vi "ProfilerTest.vi"() -> ()   [LabVIEW 2014]
uses:
  <vilib>/gmath/NI_Gmath.lvlib
panel:
  out "PositionProfile":cluster{cluster{dbl, dbl}[]}[](graph)=[{[{0.3585789582402244, 0.0}, {0.36140732971089534, -5.036567638092828e-07}, {0.36423581606672245, -9.61293257835823e-07}, {0.3670642302197405, -1.2546678051931824e-06}, {0.369892391773747, -1.1873323667103292e-06}, {0.3727209906863886, -4.852288259001522e-07}, {0.3755493268961446, 1.2019361819159102e-06}, {0.37837772838603073, 4.299709065192369e-06}, {0.38120612229890677, 9.306861087923713e-06}, {0.3840346937672675, 1.6794161055370797e-05}, {0.38686309715876277, 2.7400089421020022e-05}, {0.38969142959159164, 4.1830568179446516e-05}, {0.3925198402830219, 6.085616643129184e-05}, {0.39534837283852375, 8.530833036253735e-05}, {0.3981769428965464, 0.00011607503881997503}, {0.40100531487252966, 0.00015409536549003676}, {0.4038337851980858, 0.0002003653925144592}, {0.4066620491729108, 0.0002559183910066756}, {0.40949064017475745, 0.00032184661067566995}, {0.41231898267404327, 0.0003992561626145476}, {0.4151472322459584, 0.0004893018031565737}, {0.4179757913643334, 0.0005931795898988288}, {0.42080424013440515, 0.0007120817475880187}, {0.42363261299972726, 0.0008472339924668812}, {0.4264611387688061, 0.0009998885386174}, {0.42928945496510473, 0.0011712756792556854}, {0.4321180300590645, 0.0013626797839679785}, {0.4349463962629788, 0.0015753251147018839}, {0.43777465022828593, 0.0018104656195099959}, {0.4406032226432617, 0.0020693801641639095}, {0.4434315120502036, 0.0023532398256405924}, {0.44626009279999124, 0.0026633085947595217}, {0.4490885496571133, 0.0030007250958818303}, {0.4519170062439872, 0.0033666550409679917}, {0.45474539180496276, 0.0037622072978145747}, {0.4575737400814671, 0.004188465921919652}, {0.4604023558724684, 0.00464651952063507}, {0.4632306508066975, 0.005137264322612427}, {0.4660590176954227, 0.0056617062591942675}, {0.46888754518422093, 0.006220754083531697}, {0.47171598682256316, 0.006815191097196341}, {0.47454419326877034, 0.007445749606160159}, {0.47737285109456384, 0.008113292873994857}, {0.4802013404974829, 0.008818319578063984}, {0.4830295733801785, 0.0095613694727503}, {0.48585812789442756, 0.010343094603175375}, {0.48868640379899964, 0.011163755381214013}, {0.4915149544924278, 0.012023862733814084}, {0.49434329506372604, 0.012923544535122886}, {0.497171737305647, 0.013863094164634368}, {0.5000002749584594, 0.014842631910283946}, {0.5028286305191115, 0.015862099281043703}, {0.5056569781980829, 0.016921515585541176}, {0.5084855530715745, 0.018020855308149553}, {0.5113138558379144, 0.019159726963599216}, {0.5141422566436455, 0.020338001953235096}, {0.5169706346971762, 0.021555281125875562}, {0.5197992068851479, 0.022811235874616413}, {0.5226275593510029, 0.02410518309111191}, {0.5254560377756676, 0.025436708787521183}, {0.528284286027275, 0.026805003940692}, {0.5311127926252351, 0.02820959945311543}, {0.5339412791135189, 0.029649591762413142}, {0.5367697939830852, 0.031124175019706785}, {0.5395980099037839, 0.032632285569350675}, {0.5424265819503729, 0.03417333154853474}, {0.545255072269434, 0.03574608666415281}, {0.5480834517870963, 0.03734949267315463}, {0.5509118902564176, 0.03898256385355613}, {0.553740368824329, 0.04064417171967369}, {0.556568652677063, 0.04233302336120809}, {0.5593971125961626, 0.044048158165816725}, {0.5622256826953395, 0.04578833390525411}, {0.5650541408427635, 0.047552188047106835}, {0.5678823695638735, 0.04933840260698288}, {0.5707107335249578, 0.051145956448161785}, {0.5735393080219774, 0.05297364612388425}, {0.5763678204221673, 0.054820041534700194}, {0.5791962794223798, 0.05668389668842144}, {0.5820244134875872, 0.05856378880205473}, {0.5848531114955801, 0.06045908490205213}, {0.5876815198777922, 0.06236800907963759}, {0.590509811808415, 0.0642894935472419}, {0.5933381994308217, 0.06622252965639741}, {0.5961666861819129, 0.06816600181322202}, {0.5989949592951849, 0.07011861347290503}, {0.6018236974459827, 0.07207979542981183}, {0.6046518706223064, 0.07404784077762908}, {0.6074804451692932, 0.07602247913536116}, {0.6103087856472974, 0.07800237936364145}, {0.6131370939005591, 0.0799868514455843}, {0.6159655299441653, 0.08197523809866301}, {0.6187940939091453, 0.08396683389452729}, {0.6216224220212786, 0.08596074317195565}, {0.6244511272184643, 0.08795682791272567}, {0.6272792419089648, 0.08995390636154527}, {0.6301078589095738, 0.09195232466329135}, {0.6329362560771964, 0.09395122235875845}, {0.6357645981270923, 0.09595044178684581}, {0.6385932589450429, 0.0979500507769548}, {0.6414214187260036, 0.09994935160113598}, {1.6313712381539545, 0.7999493516011359}, {1.6370281665398847, 0.803951419959496}, {1.642684574332719, 0.8079529359236688}, {1.6483415120027398, 0.8119541698494368}, {1.6539983690163287, 0.8159539039077326}, {1.6596556635054802, 0.819951408197701}, {1.6653125310660257, 0.8239446701543608}, {1.6709694703145168, 0.8279323401920422}, {1.6766263531941783, 0.8319123326675287}, {1.682282985074101, 0.8358822305251936}, {1.6879394068533564, 0.8398395066604479}, {1.6935964190626638, 0.8437818960051781}, {1.6992532184268627, 0.8477057580086892}, {1.70491063008667, 0.8516083400146843}, {1.7105670391496792, 0.8554849779734043}, {1.7162237784800585, 0.859332821530174}, {1.7218811935075897, 0.8631481275702646}, {1.7275374178826466, 0.8669254871798622}, {1.7331945304300687, 0.870661967100665}, {1.7388514364958167, 0.8743523602708978}, {1.744508275250376, 0.8779921498769128}, {1.7501653995857358, 0.8815768325883049}, {1.7558217882719545, 0.8851009438527649}, {1.7614788664277674, 0.8885604691316429}, {1.767135829491985, 0.8919499440861656}, {1.772792234930327, 0.8952641148568315}, {1.7784493026829933, 0.8984986725061798}, {1.7841064026905955, 0.9016482200345362}, {1.7897632647477684, 0.9047076096157937}, {1.795420199823116, 0.9076720509463055}, {1.80107684483402, 0.9105364564236967}, {1.806733525727416, 0.9132961736478062}, {1.812390409338302, 0.9159465504697608}, {1.8180473081359514, 0.918482881798126}, {1.82370424507416, 0.920900699672133}, {1.8293609976576792, 0.9231955892377075}, {1.8350178638388264, 0.9253635183875473}, {1.8406748547831566, 0.9274005134168232}, {1.8463319774832216, 0.929302798916601}, {1.851988344019988, 0.9310665464586092}, {1.8576452637076741, 0.932688849389749}, {1.8633020150717972, 0.9341664072216153}, {1.8689588347334438, 0.9354964617036569}, {1.874615856039072, 0.9366764760483167}, {1.8802726191382602, 0.9377040757084186}, {1.885929833727203, 0.9385773862648643}, {1.8915861462936545, 0.9392945155796241}, {1.8972436746684436, 0.939854317274878}, {1.9028999138372154, 0.9402554507202174}, {1.9085569721805382, 0.9404972992417304}, {1.9142139634722453, 0.9405793203438549}, {1.9198707247573814, 0.9405013664325429}, {1.9255274979690329, 0.9402636012217233}, {1.9311844809276448, 0.9398664798144253}, {1.9368416418874643, 0.9393107740797157}, {1.9424982407207014, 0.9385976688034054}, {1.948154770427408, 0.9377285296837929}, {1.9538118311419879, 0.9367049472413911}, {1.959468704245492, 0.935529032771663}, {1.9651257500661143, 0.9342029930217137}, {1.9707824942395522, 0.9327295017555716}, {1.9764394982683444, 0.9311112384142088}, {1.9820960133629753, 0.9293515049839838}, {1.987753292494381, 0.9274532241336241}, {1.9934099090348023, 0.9254204232738688}, {1.99906686783999, 0.9232565214374397}, {2.0047237967048193, 0.9209656200506127}, {2.010380279393679, 0.9185520585915949}, {2.0160374263955583, 0.9160196807400908}, {2.0216939973209773, 0.9133735151338472}, {2.027350721004126, 0.910617844173485}, {2.0330078033969303, 0.9077572799132123}, {2.038664652777534, 0.904796942768744}, {2.0443217038394996, 0.9017415095326125}, {2.049978713640327, 0.8985960699865745}, {2.0556351461826123, 0.8953659381838422}, {2.0612919670827305, 0.892055588232734}, {2.066949166324256, 0.8886700317323528}, {2.072606042851228, 0.8852146891765559}, {2.0782628300431796, 0.8816943878809597}, {2.083919355872701, 0.8781141434552929}, {2.089576718776267, 0.8744780766014809}, {2.095233186517815, 0.8707920282241328}, {2.1008897971805096, 0.86705994231616}, {2.1065466194975815, 0.8632862453826441}, {2.1122035140675552, 0.8594753517073581}, {2.117860350300693, 0.8556315044422685}, {2.1235176422115813, 0.8517583212002827}, {2.129174356576727, 0.8478602789857945}, {2.1348312426096725, 0.8439404168465451}, {2.1404879039373634, 0.8400023320094359}, {2.146144651193938, 0.8360488879988732}, {2.151801616247107, 0.8320828154025052}, {2.157458635116028, 0.8281067859203439}, {2.1631152363361923, 0.8241234126529265}, {2.1687724668390422, 0.8201339534180261}, {2.174428903431, 0.8161411137841654}, {2.1800862117160427, 0.8121451197611759}, {2.185743088670165, 0.8081479874562176}, {2.1913996477159907, 0.8041504229032101}, {2.1970564563934145, 0.8001524978094131}, {3.1870059092933873, 0.10015249780941327}, {3.189834376952661, 0.09815196485448308}, {3.1926628208961687, 0.09615149471398858}, {3.195491154710077, 0.09415126670604042}, {3.198319814247035, 0.09215116912790172}, {3.2011480562768933, 0.09015200147095218}, {3.203976421854729, 0.08815373158884615}, {3.2068048663805646, 0.08615681655403101}, {3.2096333044469065, 0.08416181555271954}, {3.2124617645743654, 0.08216927872519217}, {3.215290160671209, 0.08017990602938493}, {3.2181187577501067, 0.07819421736052339}, {3.220946939449224, 0.07621341471380688}, {3.2237754858940275, 0.07423778222708795}, {3.22660380801813, 0.07226861983350559}, {3.2294323811680914, 0.07030653890209591}, {3.2322606991785543, 0.06835288293881592}, {3.2350893436336823, 0.0664082894900329}, {3.237917517860741, 0.06447438652101888}, {3.240745929431053, 0.06255180797125205}, {3.243574513512423, 0.06064175320269017}, {3.2464029865024893, 0.058745595987286174}, {3.249231234621287, 0.05686461618439337}, {3.2520597500573265, 0.05499971257506911}, {3.2548881873074937, 0.053152355156413957}, {3.25771668038416, 0.051323706706228676}, {3.260545012761648, 0.04951516151427515}, {3.2633734499117364, 0.04772780461430523}, {3.266201939035123, 0.04596292162031383}, {3.269030408345825, 0.04422179831825756}, {3.2718586604861892, 0.0425057788627582}, {3.2746872201396093, 0.040815752293008385}, {3.2775155378570093, 0.03915322950542233}, {3.280344045893975, 0.037519108419200184}, {3.28317252049387, 0.03591463984025024}, {3.2860008019498648, 0.03434099182862359}, {3.2888292025282784, 0.03279902820106029}, {3.291657898402663, 0.0312896524823099}, {3.2944861081495787, 0.029814220407712727}, {3.297314487927476, 0.02837327209971384}, {3.3001430356348505, 0.026967645470529503}, {3.302971545797128, 0.025598214957484447}, {3.305800015690742, 0.024265686411860637}, {3.308628313751244, 0.02297075698372346}, {3.311456837717748, 0.021713815872416345}, {3.3142851063333936, 0.02049557511542688}, {3.317113510341176, 0.01931628938178402}, {3.319942140639503, 0.018176278701657805}, {3.322770475473191, 0.017076025894279714}, {3.325598951730509, 0.0160155542477583}, {3.3284271585701153, 0.014995133269844946}, {3.331255650673881, 0.014014602610481333}, {3.3340842016902306, 0.013074008573941046}, {3.3369126832522826, 0.012173275404529102}, {3.3397410238060945, 0.011312224954167158}, {3.342569505843347, 0.010490497226123927}, {3.3453979692051306, 0.00970779087551378}, {3.348226168550258, 0.008963742531939212}, {3.3510547303200977, 0.00825769055905251}, {3.3538831373264912, 0.007589198022618135}, {3.356711646823256, 0.006957563668547689}, {3.359539843986255, 0.0063621701239242046}, {3.362368579114789, 0.005802072774378289}, {3.365196907570558, 0.005276630500459872}, {3.3680251947372883, 0.004784879138177739}, {3.3708538439069944, 0.00432581205227503}, {3.37368212832295, 0.00389855473132987}, {3.3765105999367697, 0.00350198195863069}, {3.3793390609903295, 0.0031350432068672773}, {3.382167341786597, 0.002796638458215678}, {3.384995900625516, 0.0024855615832211353}, {3.387824100002938, 0.0022006998955641788}, {3.3906525370972926, 0.001940785463632702}, {3.3934812447082754, 0.0017045960409560468}, {3.396309623342623, 0.0014909403278989125}, {3.399138009814577, 0.0012985386143856414}, {3.401966239444692, 0.0011261452085499501}, {3.404794884911576, 0.0009724724544487723}, {3.4076233428838814, 0.0008363048810501872}, {3.4104517350040227, 0.0007163937146592025}, {3.413279971886032, 0.0006115152322606204}, {3.416108674337413, 0.0005204426005797208}, {3.418937066744051, 0.00044202012932857693}, {3.4217652592109435, 0.00037508878451707195}, {3.424593666374727, 0.0003185198239412934}, {3.427422277158417, 0.00027123457375897997}, {3.4302507673102225, 0.0002321999436666472}, {3.4330789383343356, 0.0002004244303096675}, {3.4359075310972456, 0.00017495792053558168}, {3.4387360868980017, 0.00015491760982501435}, {3.441564460491389, 0.00013947326521591974}, {3.4443927904586418, 0.00012785381448950084}, {3.4472212072183313, 0.00011935286022231317}, {3.4500497082942103, 0.00011333131431554011}, {3.45287823807302, 0.00010921918252003449}, {3.4557064000578945, 0.00010651794748479937}, {3.458534865041683, 0.00010480148475842943}, {3.461363484864872, 0.00010371967740131771}, {3.464191891692424, 0.000102998649759517}, {3.4670201802152696, 0.00010244185295481267}, {3.469848696679472, 0.00010193103453323693}]}, {[{-0.19999989876479196, 0.0}, {-0.19599968101011692, -1.0073890062435072e-06}, {-0.19199994667744594, -1.9225945871386622e-06}, {-0.18799999265754622, -2.5093928300131422e-06}, {-0.1839997845362129, -2.374731211715307e-06}, {-0.17999974440499977, -9.705808353379095e-07}, {-0.17599979749828915, 2.403802486573782e-06}, {-0.17199988165080565, 8.599268291656234e-06}, {-0.16799989365427387, 1.8613647522725885e-05}, {-0.16399974641027576, 3.3588001121278266e-05}, {-0.1599997925054006, 5.4799691746145115e-05}, {-0.15599971752805983, 8.366224932173939e-05}, {-0.1519999497491696, 0.00012171155347277046}, {-0.14799969116464354, 0.00017061719927788325}, {-0.14399969044576694, 0.00023214732640653593}, {-0.13999981710696696, 0.00030818635937504747}, {-0.13599971002251018, 0.00040072669020160844}, {-0.13199972051983241, 0.0005118385846248636}, {-0.12799954398961128, 0.0006436933966885023}, {-0.12399969135950169, 0.0007985113946655726}, {-0.11999953380714436, 0.0009786223206733522}, {-0.11599977635493537, 0.0011863568434762873}, {-0.11199968221715566, 0.0014241648800392122}, {-0.1079995336266278, 0.0016944857648968758}, {-0.1039995400032736, 0.001999785318751084}, {-0.0999995485779444, 0.0023425740446704636}, {-0.09599988630439422, 0.002725329666204823}, {-0.09199964994606155, 0.003150653182229347}, {-0.0879995735663378, 0.003620974170090313}, {-0.08399980405477737, 0.004138748410156852}, {-0.07999999916436557, 0.004706466584627505}, {-0.0759998629865118, 0.005326589855729003}, {-0.07199961765286897, 0.006001456251807512}, {-0.06799979603645853, 0.006733274802642866}, {-0.06399986297303943, 0.007524374874632924}, {-0.05999988752456636, 0.008376908350246326}, {-0.05599990000907039, 0.009292947639581864}, {-0.05199983599363788, 0.01027449455001387}, {-0.0479997168866717, 0.011323431486463826}, {-0.043999880594600596, 0.012441440279665605}, {-0.03999975405466372, 0.013630342589506319}, {-0.0359996009332965, 0.014891608226232011}, {-0.0319998496375525, 0.016226503794618343}, {-0.027999840689221626, 0.017636524080817256}, {-0.023999769484300045, 0.01912274965632081}, {-0.019999859236598534, 0.02068609238390031}, {-0.015999581163923807, 0.022327615932514405}, {-0.011999560949191997, 0.024047767634961383}, {-0.007999627735662542, 0.0258471587522783}, {-0.003999840056932571, 0.027726148951964028}, {4.1224803332798345e-08, 0.029685085391621735}, {0.004000050239789517, 0.031724070314499614}, {0.008000456453749596, 0.03384317789924717}, {0.012000279308808297, 0.036041646730799924}, {0.01600045667166006, 0.03831959245048956}, {0.020000319536075086, 0.0406760872990872}, {0.024000111618094132, 0.043110562715697}, {0.028000225990225294, 0.04562241437367817}, {0.032000049999004576, 0.048210260902798945}, {0.03600008512101396, 0.0508732840581242}, {0.04000039271398916, 0.05361025939014283}, {0.044000091642358304, 0.05641916285666922}, {0.048000181014672, 0.059299150534354306}, {0.05200011351256987, 0.062248173384726865}, {0.056000112327799806, 0.06526461734444017}, {0.06000022144401757, 0.06834663565227124}, {0.064000383055079, 0.07149220267414197}, {0.06800031247824058, 0.07469901258558052}, {0.07200034033342433, 0.07796516512426935}, {0.07600027932901354, 0.08128826939114384}, {0.08000026425003828, 0.08466613105003873}, {0.0840001923497527, 0.08809629967990842}, {0.0880003922731866, 0.09157664885847029}, {0.0920002782494199, 0.0951042166523484}, {0.09600047961452424, 0.09867707678906977}, {0.10000000532914792, 0.10229183759674812}, {0.10400001306758956, 0.10594703169374545}, {0.10800036848861945, 0.1096400376566363}, {0.11200032981283371, 0.11336766901734488}, {0.11600008949348195, 0.11712761642391986}, {0.12000007493219605, 0.12091783055886571}, {0.12400034372560143, 0.1247359592065738}, {0.12800032101307562, 0.1285790899697627}, {0.13200010382857721, 0.1324450062315782}, {0.136000282340795, 0.136332041830554}, {0.140000107015834, 0.1402373066816576}, {0.14400010015815898, 0.14415923185061982}, {0.14800022290551634, 0.14809579610572363}, {0.15200043336748306, 0.15204507487706104}, {0.15600046519792107, 0.15600502838951402}, {0.16000030990992947, 0.15997398560380838}, {0.16400028639019507, 0.16395072318406365}, {0.16800034270890934, 0.16793377813693242}, {0.17200018742098142, 0.1719215813066752}, {0.17600029908556936, 0.1759134694582433}, {0.18000030977545484, 0.17990807800480932}, {0.18400043689948456, 0.18390477310907577}, {0.18800042429414585, 0.18790259797400644}, {0.19200038479082773, 0.1919011173282485}, {0.19600040771091862, 0.1959000275178594}, {0.20000004677832364, 0.19989864599950807}, {0.4414214002333889, 0.44132000223681755}, {0.4425930563548353, 0.44249174477995745}, {0.44376451083174406, 0.44366327776622694}, {0.4449361528206526, 0.44483497009649164}, {0.44610773574002566, 0.4460065414606963}, {0.4472792694650633, 0.44717795473398797}, {0.4484508146081704, 0.4483492104091164}, {0.4496225058954555, 0.44952037013522933}, {0.4507940466763791, 0.450691051809895}, {0.45196552872069967, 0.4518612494012046}, {0.45313714814505635, 0.45303104906957864}, {0.45430870800618584, 0.4542001329972505}, {0.455480368486206, 0.4553685288935537}, {0.4566518320526547, 0.45653579765596497}, {0.4578234266226369, 0.45770211372784}, {0.45899499073062155, 0.45886715458815225}, {0.4601665696585886, 0.46003079501259997}, {0.4613382066626694, 0.4611928995789317}, {0.46250980465709973, 0.4623531864472321}, {0.4636813333148966, 0.46351143382539056}, {0.46485294696082025, 0.4646675964660735}, {0.46602440998324857, 0.46582123931988156}, {0.4671960103661306, 0.46697243909305663}, {0.4683675673018719, 0.4681208075153042}, {0.4695392113563284, 0.4692662595439}, {0.4707106821148058, 0.47040832639914043}, {0.4718822981449211, 0.4715471033725848}, {0.47305394571359355, 0.4726822637245265}, {0.4742254015820826, 0.47381337739933127}, {0.475397014001019, 0.4749405679832672}, {0.4765685434857642, 0.4760633943946943}, {0.47774024306100515, 0.4771818916827408}, {0.47891171261257387, 0.47829547550435225}, {0.480083269082721, 0.4794042502387827}, {0.4812549326403847, 0.480508041729458}, {0.4824264162590043, 0.48160639457731486}, {0.4835980290984438, 0.4826994207461059}, {0.48476959934296643, 0.4837867890638945}, {0.48594119639124184, 0.48486840240009016}, {0.4871127014588357, 0.48594399920929526}, {0.4882843839237273, 0.48701368363768904}, {0.48945586984689426, 0.4880769823776956}, {0.4906274495843984, 0.4891340386619428}, {0.49179905695308623, 0.49018468209207416}, {0.4929705646527205, 0.4912287012783078}, {0.49414213910265375, 0.4922661592233995}, {0.4953137471707906, 0.493296952737306}, {0.4964853379325727, 0.4943209767511561}, {0.4976569412605734, 0.49533821040362036}, {0.49882846385056656, 0.4963485395687738}, {0.5000001007577792, 0.49735211188887296}, {0.5011717107493813, 0.49834879885449046}, {0.5023431819019044, 0.4993385134777973}, {0.503514804291589, 0.5003215210017554}, {0.5046863878897527, 0.5012976947188631}, {0.5058578771874219, 0.5022670365425134}, {0.507029449302316, 0.5032297532462725}, {0.5082010843849928, 0.5041859002731838}, {0.5093726385054977, 0.5051354459039696}, {0.5105441823005161, 0.5060785459842273}, {0.5117158470243144, 0.5070154149740866}, {0.5128873409953718, 0.5079459411678274}, {0.5140589482240441, 0.5088704826980944}, {0.5152304955977388, 0.5097890450494283}, {0.5164021051280252, 0.51070187625702}, {0.5175736650703935, 0.5116090508129194}, {0.5187452066112065, 0.5125107636242076}, {0.5199167705315969, 0.5134072242794286}, {0.521088447950074, 0.5142986871006676}, {0.5222599400133885, 0.5151851171755801}, {0.523431563162278, 0.5160669520696957}, {0.5246030584245023, 0.5169441995821659}, {0.525774645188754, 0.5178172311444779}, {0.5269462743681366, 0.5186862197686207}, {0.5281177626827985, 0.5195512428574444}, {0.5292894081179139, 0.5204127349188776}, {0.5304610201524012, 0.5212707706994473}, {0.5316324930917736, 0.5221254889199889}, {0.5328041519745816, 0.5229773410969261}, {0.5339756720532917, 0.5238263037766439}, {0.5351473133352743, 0.5246727757690263}, {0.5363188878545998, 0.5255168280441613}, {0.5374903746929753, 0.5263586487354304}, {0.5386619789837332, 0.5271985829392737}, {0.5398335106914113, 0.5280366863016444}, {0.5410051293976712, 0.5288732584507841}, {0.5421767169633624, 0.5297083931596693}, {0.5433482619153063, 0.5305422526568511}, {0.5445198030072892, 0.5313750262365045}, {0.5456914727468875, 0.532206960314916}, {0.5468629710622596, 0.5330379843825885}, {0.5480345111614261, 0.533868381883265}, {0.5492061255068107, 0.534698296859006}, {0.5503777415694471, 0.5355277875883844}, {0.5515492929101521, 0.5363569049019212}, {0.5527208277775615, 0.5371857685582488}, {0.553892450538768, 0.5380145253750436}, {0.5550639609523547, 0.5388430938322217}, {0.556235622140303, 0.5396717070351608}, {0.5574071803271078, 0.5405002192179884}, {0.5585787661569405, 0.5413287430532149}, {0.9242643273297185, 0.7999073868159052}, {0.929921548524073, 0.8039096623225616}, {0.9355784215761808, 0.8079115073821405}, {0.9412350013369843, 0.8119124880397954}, {0.9468921630436015, 0.8159124373092295}, {0.9525486904380175, 0.819909399346364}, {0.9582052015784316, 0.8239024098368071}, {0.9638621409444782, 0.8278900803412275}, {0.9695195002205597, 0.8318704081179266}, {0.9751760758083804, 0.8358402662368315}, {0.9808327618496375, 0.8397977266953995}, {0.9864898137531176, 0.8437401425881922}, {0.9921463947473637, 0.8476638521197739}, {0.9978032170525506, 0.8515660280998896}, {1.003460530752386, 0.8554432858158529}, {1.009116911187835, 0.8592908835559361}, {1.0147741193506303, 0.8631060499197625}, {1.0204308755409022, 0.8668837633226054}, {1.0260876727861046, 0.8706200326926197}, {1.0317447954655272, 0.874310565022905}, {1.0374015661432985, 0.8779503077920353}, {1.043058137682256, 0.8815346401110078}, {1.0487150240955871, 0.8850590615836236}, {1.0543719043665345, 0.88851846422959}, {1.060029096589934, 0.8919080745181172}, {1.065685429439742, 0.8952221996022159}, {1.0713425964214403, 0.8984568104196354}, {1.0769992033567934, 0.9016060827397802}, {1.0826560559146963, 0.9046654705218566}, {1.0883129589417313, 0.9076298989337609}, {1.0939702205149247, 0.910494615362273}, {1.0996265598753132, 0.9132541621078781}, {1.105283836955477, 0.9159047186902207}, {1.1109403760089414, 0.91844088365343}, {1.1165971995481687, 0.9208586528286369}, {1.1222544782517372, 0.9231537509981205}, {1.1279114432072874, 0.9253217059080077}, {1.1335681841002707, 0.9273586002378953}, {1.1392247861666531, 0.9292607090290489}, {1.1448818235678626, 0.9310246621579363}, {1.1505383759100252, 0.9326468522680382}, {1.1561953985345024, 0.9341244745390975}, {1.1618524255153602, 0.9354545649410907}, {1.1675093456998005, 0.9366345437498719}, {1.1731659459051444, 0.9376621027538383}, {1.1788230564772095, 0.9385353897143254}, {1.1844798839672763, 0.9392525709908157}, {1.1901362907240176, 0.9398122567807516}, {1.1957932753027172, 0.9402134433969267}, {1.201450090819772, 0.9404552747648737}, {1.2071071216023228, 0.940537292526543}, {1.212764198400767, 0.9404593253359443}, {1.2184208905746234, 0.940221551308664}, {1.224077437366832, 0.9398244556101041}, {1.2297343484728858, 0.93926877912245}, {1.2353910937950443, 0.9385556614849903}, {1.2410482682276731, 0.9376864185025636}, {1.2467047694266284, 0.9366629313691335}, {1.252362292016941, 0.9354868748756813}, {1.2580190496423298, 0.934160890995147}, {1.2636756820776487, 0.9326874225339583}, {1.269332769855172, 0.9310691294235703}, {1.2749896884922032, 0.9293092587566079}, {1.2806464505494892, 0.9274111413250792}, {1.2863032582273766, 0.9253782658291371}, {1.291959951392885, 0.9232144606547501}, {1.2976166036160062, 0.9209236724930789}, {1.3032736382140597, 0.9185098738070043}, {1.3089308303349438, 0.9159774679191098}, {1.3145874344345478, 0.913331278487835}, {1.3202443034399853, 0.9105755270929005}, {1.325900911772757, 0.9077151962653593}, {1.3315576359281633, 0.904754923856247}, {1.337214672487806, 0.9016994988460685}, {1.3428714181662182, 0.8985542086676657}, {1.3485282661068558, 0.8953238409608435}, {1.3541851823106972, 0.892013432949929}, {1.3598419628607776, 0.8886281269096362}, {1.3654990246978953, 0.8851726724979577}, {1.371155759594115, 0.8816524042328363}, {1.376813028367411, 0.8780716865509465}, {1.382469316372244, 0.8744363092119464}, {1.3881267941373372, 0.8707496018444171}, {1.393783607066272, 0.8670173770262329}, {1.3994402323440995, 0.8632438065863061}, {1.4050970950300925, 0.8594329306909564}, {1.4107541106681898, 0.8555889578573352}, {1.4164106754402872, 0.8517162704989582}, {1.4220678305277044, 0.8478179235549277}, {1.4277245441984887, 0.843898179472249}, {1.4333813095525862, 0.8399600211681962}, {1.4390382421719268, 0.8360064463976294}, {1.4446948425287693, 0.832040628668918}, {1.4503518872688121, 0.8280645806348984}, {1.456008858576261, 0.8240809462537876}, {1.4616655418021376, 0.8200918726507659}, {1.4673226620027124, 0.8160985502414425}, {1.4729794006569625, 0.8121029584009362}, {1.4786364261680085, 0.8081057210813869}, {1.4842927889334165, 0.8041082952253847}, {1.4899498677677236, 0.8001101791974354}]}]
  out "VelocityProfile":T1(graph)=[{[{"Time"=0.0, "delVelocity"=0.0}, {"Time"=0.5, "delVelocity"=0.0}, {"Time"=0.5, "delVelocity"=0.7071067811865475}, {"Time"=1.2071067811865475, "delVelocity"=0.7071067811865475}, {"Time"=1.2071067811865475, "delVelocity"=0.7071067811865475}, {"Time"=1.914213562373095, "delVelocity"=0.7071067811865475}, {"Time"=1.914213562373095, "delVelocity"=-0.7071067811865475}, {"Time"=2.6213203435596424, "delVelocity"=-0.7071067811865475}, {"Time"=2.6213203435596424, "delVelocity"=-0.7071067811865475}, {"Time"=3.32842712474619, "delVelocity"=-0.7071067811865475}, {"Time"=3.32842712474619, "delVelocity"=0.0}, {"Time"=3.82842712474619, "delVelocity"=0.0}]}, {[{"Time"=0.0, "delVelocity"=1.0}, {"Time"=0.5, "delVelocity"=1.0}, {"Time"=0.5, "delVelocity"=0.7071067811865475}, {"Time"=1.2071067811865475, "delVelocity"=0.7071067811865475}, {"Time"=1.2071067811865475, "delVelocity"=-0.7071067811865475}, {"Time"=1.914213562373095, "delVelocity"=-0.7071067811865475}, {"Time"=1.914213562373095, "delVelocity"=-0.7071067811865475}, {"Time"=2.6213203435596424, "delVelocity"=-0.7071067811865475}, {"Time"=2.6213203435596424, "delVelocity"=0.7071067811865475}, {"Time"=3.32842712474619, "delVelocity"=0.7071067811865475}, {"Time"=3.32842712474619, "delVelocity"=-1.0}, {"Time"=3.82842712474619, "delVelocity"=-1.0}]}, {[{"Time"=0.3585789372997002, "delVelocity"=-0.0001792365071832489}, {"Time"=0.3614071545552001, "delVelocity"=-0.00017458441517853346}, {"Time"=0.36423572893526784, "delVelocity"=-0.00014204063846811398}, {"Time"=0.3670639632118197, "delVelocity"=-5.383805665773475e-05}, {"Time"=0.36989264114898573, "delVelocity"=0.00011761237296677458}, {"Time"=0.37272091614121855, "delVelocity"=0.00039948953704023796}, {"Time"=0.3755494647516993, "delVelocity"=0.0008186487665399644}, {"Time"=0.3783777473285121, "delVelocity"=0.0014012607664726793}, {"Time"=0.3812061229225435, "delVelocity"=0.0021729897805010103}, {"Time"=0.38403470454106864, "delVelocity"=0.0031587588564301935}, {"Time"=0.3868629977834092, "delVelocity"=0.004382401324505711}, {"Time"=0.38969136917972663, "delVelocity"=0.005867124810335461}, {"Time"=0.39251979277144244, "delVelocity"=0.007634979593229136}, {"Time"=0.39534838845493514, "delVelocity"=0.009707005740472298}, {"Time"=0.39817681548017336, "delVelocity"=0.012102684586240824}, {"Time"=0.40100534457872006, "delVelocity"=0.014840687222719614}, {"Time"=0.4038336633426032, "delVelocity"=0.0179377919352845}, {"Time"=0.4066620347350509, "delVelocity"=0.02140993871458358}, {"Time"=0.40949059848971625, "delVelocity"=0.02527155165874137}, {"Time"=0.41231906902213483, "delVelocity"=0.02953492910242824}, {"Time"=0.41514727880065005, "delVelocity"=0.034210822821049536}, {"Time"=0.4179757697137227, "delVelocity"=0.03930958425494159}, {"Time"=0.4208041505975349, "delVelocity"=0.044838330538051065}, {"Time"=0.42363274041297005, "delVelocity"=0.05080379479086151}, {"Time"=0.4264609446485784, "delVelocity"=0.05720904657277652}, {"Time"=0.42928948083587415, "delVelocity"=0.06405832415156026}, {"Time"=0.4321179104931776, "delVelocity"=0.07135149505678157}, {"Time"=0.4349462898055023, "delVelocity"=0.07908779073780743}, {"Time"=0.43777492555641156, "delVelocity"=0.08726547255299479}, {"Time"=0.440603184307256, "delVelocity"=0.09587831636816485}, {"Time"=0.4434315742170515, "delVelocity"=0.10492172641799466}, {"Time"=0.4462601755011201, "delVelocity"=0.11438825223363258}, {"Time"=0.44908845794333163, "delVelocity"=0.12426664423888009}, {"Time"=0.4519169670827088, "delVelocity"=0.13454770611698755}, {"Time"=0.45474521196459666, "delVelocity"=0.14521697954990498}, {"Time"=0.4575739003025374, "delVelocity"=0.15626296631627415}, {"Time"=0.46040213473682384, "delVelocity"=0.16766647808868268}, {"Time"=0.46323062024803036, "delVelocity"=0.17941321729618565}, {"Time"=0.4660589612526859, "delVelocity"=0.19148310975378835}, {"Time"=0.4688873570337898, "delVelocity"=0.20385726174041544}, {"Time"=0.47171603193767353, "delVelocity"=0.21651577622337057}, {"Time"=0.4745443064308536, "delVelocity"=0.22943354797582302}, {"Time"=0.4773728359515352, "delVelocity"=0.24259047232369207}, {"Time"=0.48020127129538714, "delVelocity"=0.2559609285936483}, {"Time"=0.4830294665719006, "delVelocity"=0.26951933195701544}, {"Time"=0.48585804709742214, "delVelocity"=0.28324308698307255}, {"Time"=0.48868659130779746, "delVelocity"=0.2971039239168765}, {"Time"=0.4915148367169637, "delVelocity"=0.3110737400057257}, {"Time"=0.4943431686818007, "delVelocity"=0.3251271992669252}, {"Time"=0.49717167854772326, "delVelocity"=0.33923720895526754}, {"Time"=0.5000000546972132, "delVelocity"=0.3533744385664503}, {"Time"=0.5028284821670278, "delVelocity"=0.36751192398643623}, {"Time"=0.5056571129731147, "delVelocity"=0.38162253361585663}, {"Time"=0.5084855100041511, "delVelocity"=0.3956763084069582}, {"Time"=0.5113138207874259, "delVelocity"=0.4096464343537216}, {"Time"=0.5141423876906802, "delVelocity"=0.42350736391784144}, {"Time"=0.5169706883749067, "delVelocity"=0.4372297457353656}, {"Time"=0.5197990473550455, "delVelocity"=0.4507889190028031}, {"Time"=0.5226276041846981, "delVelocity"=0.46415992241385895}, {"Time"=0.5254559733793619, "delVelocity"=0.4773160723395265}, {"Time"=0.528284485539743, "delVelocity"=0.49023489425176575}, {"Time"=0.5311130032027764, "delVelocity"=0.5028926629278029}, {"Time"=0.5339412202627203, "delVelocity"=0.5152660049930666}, {"Time"=0.5367698274829419, "delVelocity"=0.5273369984234632}, {"Time"=0.5395981398460561, "delVelocity"=0.5390829760933195}, {"Time"=0.5424265970295017, "delVelocity"=0.5504873379870242}, {"Time"=0.5452551451238262, "delVelocity"=0.5615327216735874}, {"Time"=0.54808344388221, "delVelocity"=0.5722021464162114}, {"Time"=0.5509119179105609, "delVelocity"=0.5824830256328718}, {"Time"=0.5537404129526612, "delVelocity"=0.5923620906222508}, {"Time"=0.5565687779440852, "delVelocity"=0.6018277562039842}, {"Time"=0.5593972583245639, "delVelocity"=0.6108713955657362}, {"Time"=0.5622256841039776, "delVelocity"=0.619484667356805}, {"Time"=0.565053950716157, "delVelocity"=0.6276612160904423}, {"Time"=0.5678824573267028, "delVelocity"=0.6353978123922776}, {"Time"=0.5707108617800417, "delVelocity"=0.6426908625488048}, {"Time"=0.5735394105328995, "delVelocity"=0.649540115784144}, {"Time"=0.5763677859838527, "delVelocity"=0.655945686424771}, {"Time"=0.5791962246140434, "delVelocity"=0.6619107618810302}, {"Time"=0.5820246423408068, "delVelocity"=0.6674395198566198}, {"Time"=0.5848528293305703, "delVelocity"=0.6725376941320429}, {"Time"=0.5876814801968644, "delVelocity"=0.6772142686544201}, {"Time"=0.5905097113576887, "delVelocity"=0.6814772233057991}, {"Time"=0.5933382563833661, "delVelocity"=0.6853387686236289}, {"Time"=0.596166551519606, "delVelocity"=0.6888107875595025}, {"Time"=0.5989952324211197, "delVelocity"=0.6919082375578784}, {"Time"=0.6018233933045567, "delVelocity"=0.6946458348261745}, {"Time"=0.604652115988389, "delVelocity"=0.6970417222394006}, {"Time"=0.6074803538352285, "delVelocity"=0.6991134499047988}, {"Time"=0.6103088388424633, "delVelocity"=0.7008813246957363}, {"Time"=0.6131371065355488, "delVelocity"=0.7023659786442497}, {"Time"=0.6159658179844651, "delVelocity"=0.7035897746602853}, {"Time"=0.6187939759452719, "delVelocity"=0.704575370953532}, {"Time"=0.62162252022806, "delVelocity"=0.7053471330545619}, {"Time"=0.6244509031661403, "delVelocity"=0.7059297459860256}, {"Time"=0.6272794165414343, "delVelocity"=0.7063488813302021}, {"Time"=0.6301078168145527, "delVelocity"=0.7066307537576233}, {"Time"=0.6329361502130386, "delVelocity"=0.7068021732400744}, {"Time"=0.6357647778627531, "delVelocity"=0.7068903807898067}, {"Time"=0.6385931101996192, "delVelocity"=0.706922915881989}, {"Time"=0.6414216446130907, "delVelocity"=0.7069275666679519}, {"Time"=1.6313708605192776, "delVelocity"=0.7074652541686401}, {"Time"=1.6370283289657213, "delVelocity"=0.70745595001063}, {"Time"=1.64268505210938, "delVelocity"=0.7073908709190725}, {"Time"=1.6483419005861701, "delVelocity"=0.7072144594942864}, {"Time"=1.6539985339341796, "delVelocity"=0.7068716170809686}, {"Time"=1.6596553573044943, "delVelocity"=0.7063078631064793}, {"Time"=1.6653123659636604, "delVelocity"=0.7054695866707046}, {"Time"=1.6709690722525936, "delVelocity"=0.7043043656203191}, {"Time"=1.6766257701071108, "delVelocity"=0.7027609557446964}, {"Time"=1.6822825652628008, "delVelocity"=0.7007896005668409}, {"Time"=1.6879394368577818, "delVelocity"=0.6983422558120453}, {"Time"=1.6935967713559423, "delVelocity"=0.6953725250871411}, {"Time"=1.6992531410747387, "delVelocity"=0.6918371376486618}, {"Time"=1.7049100974502591, "delVelocity"=0.6876933221587315}, {"Time"=1.7105670938400341, "delVelocity"=0.68290191768123}, {"Time"=1.7162242217258903, "delVelocity"=0.6774259094922764}, {"Time"=1.7218805298735567, "delVelocity"=0.6712321452859737}, {"Time"=1.7275379183767092, "delVelocity"=0.66428712514733}, {"Time"=1.7331943065517328, "delVelocity"=0.6565649840723321}, {"Time"=1.7388511368323198, "delVelocity"=0.6480385348463364}, {"Time"=1.7445083714898828, "delVelocity"=0.6386854895981801}, {"Time"=1.750165383494738, "delVelocity"=0.628487940381774}, {"Time"=1.7558220098174375, "delVelocity"=0.617430749102444}, {"Time"=1.761478597836572, "delVelocity"=0.6055011616275979}, {"Time"=1.7671357795996112, "delVelocity"=0.5926889863919105}, {"Time"=1.772792533798002, "delVelocity"=0.5789912459345068}, {"Time"=1.7784495953059327, "delVelocity"=0.5644044360260807}, {"Time"=1.7841063743048422, "delVelocity"=0.5489318245018641}, {"Time"=1.7897631680944068, "delVelocity"=0.5325779125677164}, {"Time"=1.7954202783434177, "delVelocity"=0.5153504809040148}, {"Time"=1.8010769676524259, "delVelocity"=0.4972639721933123}, {"Time"=1.8067338436870652, "delVelocity"=0.4783320655935046}, {"Time"=1.8123907114525146, "delVelocity"=0.4585742764569548}, {"Time"=1.818047105323491, "delVelocity"=0.4380144956019353}, {"Time"=1.8237038983991487, "delVelocity"=0.4166748973282096}, {"Time"=1.829361050958994, "delVelocity"=0.3945838827119952}, {"Time"=1.8350181586000462, "delVelocity"=0.37177433825550243}, {"Time"=1.8406747569478197, "delVelocity"=0.348282443183084}, {"Time"=1.846331858523024, "delVelocity"=0.32414089913353644}, {"Time"=1.8519882556678715, "delVelocity"=0.2993943482159402}, {"Time"=1.8576454890560687, "delVelocity"=0.27407789040683306}, {"Time"=1.8633022279196483, "delVelocity"=0.24824152258086585}, {"Time"=1.868959355544059, "delVelocity"=0.22192738330028555}, {"Time"=1.8746156547825092, "delVelocity"=0.19518921486911434}, {"Time"=1.8802727418460994, "delVelocity"=0.1680691034498677}, {"Time"=1.8859298165234244, "delVelocity"=0.140622025024852}, {"Time"=1.8915861623851267, "delVelocity"=0.11290401789787008}, {"Time"=1.897243429058919, "delVelocity"=0.08496057581352412}, {"Time"=1.9029001706167825, "delVelocity"=0.056853276715967516}, {"Time"=1.9085573671622793, "delVelocity"=0.028632376619533995}, {"Time"=1.914213810538259, "delVelocity"=0.0003594619641865693}, {"Time"=1.9198710022976708, "delVelocity"=-0.02791719278573379}, {"Time"=1.9255275472202735, "delVelocity"=-0.05613484215261444}, {"Time"=1.9311844769472493, "delVelocity"=-0.08424308069560826}, {"Time"=1.9368413324862481, "delVelocity"=-0.11218450261823398}, {"Time"=1.942498466297604, "delVelocity"=-0.1399063752132811}, {"Time"=1.9481548045013446, "delVelocity"=-0.16734988551838936}, {"Time"=1.953811723823739, "delVelocity"=-0.1944692264394997}, {"Time"=1.9594689992350212, "delVelocity"=-0.2212120181752636}, {"Time"=1.9651252700757245, "delVelocity"=-0.2475221786157955}, {"Time"=1.9707825699253025, "delVelocity"=-0.2733611278416268}, {"Time"=1.9764391409619435, "delVelocity"=-0.29867464821825074}, {"Time"=1.9820962923189342, "delVelocity"=-0.32342452182519454}, {"Time"=1.9877533093356374, "delVelocity"=-0.3475656930159017}, {"Time"=1.9934098649386587, "delVelocity"=-0.37105740530169196}, {"Time"=1.9990663881252595, "delVelocity"=-0.39386462686489154}, {"Time"=2.0047238522544375, "delVelocity"=-0.41595691063682616}, {"Time"=2.010380457753478, "delVelocity"=-0.4372958477619042}, {"Time"=2.0160371070934664, "delVelocity"=-0.45785660036174947}, {"Time"=2.021694148656956, "delVelocity"=-0.4776150100966974}, {"Time"=2.0273510057292996, "delVelocity"=-0.49654685577287405}, {"Time"=2.033008170735235, "delVelocity"=-0.5146348534928147}, {"Time"=2.038664392754307, "delVelocity"=-0.5318595796545946}, {"Time"=2.0443216312875054, "delVelocity"=-0.5482148109240403}, {"Time"=2.0499787368780273, "delVelocity"=-0.5636882893193209}, {"Time"=2.055635454997253, "delVelocity"=-0.5782741886117173}, {"Time"=2.0612923517192776, "delVelocity"=-0.5919722647639112}, {"Time"=2.066949087214947, "delVelocity"=-0.6047834436308521}, {"Time"=2.072605689360835, "delVelocity"=-0.6167131086575173}, {"Time"=2.078262467320261, "delVelocity"=-0.6277706308594238}, {"Time"=2.083919264213326, "delVelocity"=-0.6379678309783434}, {"Time"=2.0895760585375887, "delVelocity"=-0.6473202344701585}, {"Time"=2.095233216774404, "delVelocity"=-0.6558472704729164}, {"Time"=2.1008900282072034, "delVelocity"=-0.6635700266294788}, {"Time"=2.106546890230187, "delVelocity"=-0.6705144430462511}, {"Time"=2.112203570583902, "delVelocity"=-0.6767086661479065}, {"Time"=2.1178603707872914, "delVelocity"=-0.6821844030858735}, {"Time"=2.1235177973198405, "delVelocity"=-0.686976209860622}, {"Time"=2.1291742835806526, "delVelocity"=-0.6911197184979423}, {"Time"=2.1348314158663633, "delVelocity"=-0.6946556031887143}, {"Time"=2.14048811042124, "delVelocity"=-0.6976250103473816}, {"Time"=2.1461449724401507, "delVelocity"=-0.7000723913403561}, {"Time"=2.1518018488638933, "delVelocity"=-0.7020438086077725}, {"Time"=2.1574585226944065, "delVelocity"=-0.7035872399341707}, {"Time"=2.163115527199548, "delVelocity"=-0.7047525386036149}, {"Time"=2.168772310614422, "delVelocity"=-0.7055907931626493}, {"Time"=2.174428913678485, "delVelocity"=-0.7061545443840036}, {"Time"=2.1800858898241153, "delVelocity"=-0.706497420902148}, {"Time"=2.1857426652641214, "delVelocity"=-0.7066738360364466}, {"Time"=2.19139987061549, "delVelocity"=-0.7067389216842634}, {"Time"=2.1970564289360173, "delVelocity"=-0.7067482248576793}, {"Time"=3.187005784138076, "delVelocity"=-0.7072860176937305}, {"Time"=3.189834288350992, "delVelocity"=-0.7072813649416156}, {"Time"=3.192662808771445, "delVelocity"=-0.7072488202510316}, {"Time"=3.1954910580349534, "delVelocity"=-0.7071606150441714}, {"Time"=3.1983197624857014, "delVelocity"=-0.7069891592829485}, {"Time"=3.201147965238078, "delVelocity"=-0.7067072856419387}, {"Time"=3.2039766246600223, "delVelocity"=-0.7062881043455776}, {"Time"=3.206804849882162, "delVelocity"=-0.705705496018832}, {"Time"=3.209633519184075, "delVelocity"=-0.7049336688659867}, {"Time"=3.212461949520872, "delVelocity"=-0.7039479269863322}, {"Time"=3.2152902239392955, "delVelocity"=-0.7027242718807426}, {"Time"=3.218118803183533, "delVelocity"=-0.7012394073770938}, {"Time"=3.220947227292184, "delVelocity"=-0.6994715071674029}, {"Time"=3.2237754254808766, "delVelocity"=-0.697399746245904}, {"Time"=3.226603776803699, "delVelocity"=-0.6950041316585017}, {"Time"=3.229432358373043, "delVelocity"=-0.6922660797480806}, {"Time"=3.2322609188146774, "delVelocity"=-0.6891686927892459}, {"Time"=3.2350890581295912, "delVelocity"=-0.6856968121614636}, {"Time"=3.2379177092921245, "delVelocity"=-0.6818350704634044}, {"Time"=3.240745900166992, "delVelocity"=-0.6775721188246555}, {"Time"=3.243574341285707, "delVelocity"=-0.6728958504247995}, {"Time"=3.246402769179822, "delVelocity"=-0.6677971979344232}, {"Time"=3.2492312582924536, "delVelocity"=-0.6622682318602605}, {"Time"=3.25205989201715, "delVelocity"=-0.6563026548849106}, {"Time"=3.254888094776546, "delVelocity"=-0.6498973828593262}, {"Time"=3.257716741281851, "delVelocity"=-0.6430478059158314}, {"Time"=3.2605452003419253, "delVelocity"=-0.6357545160035568}, {"Time"=3.2633736104056608, "delVelocity"=-0.6280180884888316}, {"Time"=3.2662017572421447, "delVelocity"=-0.6198418082687958}, {"Time"=3.269030455734668, "delVelocity"=-0.6112276174924648}, {"Time"=3.27185881575975, "delVelocity"=-0.6021842643067579}, {"Time"=3.274687064599734, "delVelocity"=-0.592718908271546}, {"Time"=3.277515760604426, "delVelocity"=-0.5828390581233165}, {"Time"=3.2803441544575356, "delVelocity"=-0.5725583809582662}, {"Time"=3.2831723147720164, "delVelocity"=-0.5618894069001911}, {"Time"=3.286001043707234, "delVelocity"=-0.5508432456281673}, {"Time"=3.2888294591249103, "delVelocity"=-0.5394389751919199}, {"Time"=3.2916577898699693, "delVelocity"=-0.5276928495482189}, {"Time"=3.294486025222602, "delVelocity"=-0.5156233949275233}, {"Time"=3.29731443994446, "delVelocity"=-0.5032491524597454}, {"Time"=3.300143127332278, "delVelocity"=-0.4905905735359304}, {"Time"=3.302971463377366, "delVelocity"=-0.47767250955756196}, {"Time"=3.3057998005209885, "delVelocity"=-0.4645164750595071}, {"Time"=3.30862830134805, "delVelocity"=-0.45114570947988925}, {"Time"=3.3114567730720634, "delVelocity"=-0.4375859705363665}, {"Time"=3.3142852702660077, "delVelocity"=-0.423862605666038}, {"Time"=3.317113630116878, "delVelocity"=-0.41000266627224224}, {"Time"=3.3199418855542673, "delVelocity"=-0.39603279915683914}, {"Time"=3.3227704290566797, "delVelocity"=-0.3819782851777837}, {"Time"=3.325598858341502, "delVelocity"=-0.36786867414921726}, {"Time"=3.32842730781108, "delVelocity"=-0.3537310770507615}, {"Time"=3.3312556127148967, "delVelocity"=-0.33959420510483745}, {"Time"=3.3340840017818767, "delVelocity"=-0.3254848013347841}, {"Time"=3.3369127036442525, "delVelocity"=-0.3114295131544838}, {"Time"=3.339740881847436, "delVelocity"=-0.29746004632867723}, {"Time"=3.342569505708803, "delVelocity"=-0.2835988416192666}, {"Time"=3.345397871716808, "delVelocity"=-0.26987615092977024}, {"Time"=3.3482261815980103, "delVelocity"=-0.25631722291006054}, {"Time"=3.351054753059134, "delVelocity"=-0.24294616043848144}, {"Time"=3.3538831083022074, "delVelocity"=-0.22979008674287787}, {"Time"=3.356711529678838, "delVelocity"=-0.2168716873141901}, {"Time"=3.3595398807518286, "delVelocity"=-0.2042146602602547}, {"Time"=3.362368497955865, "delVelocity"=-0.19183957588909795}, {"Time"=3.36519689042299, "delVelocity"=-0.1797695177001717}, {"Time"=3.3680254031970507, "delVelocity"=-0.16802272705341192}, {"Time"=3.3708535819952568, "delVelocity"=-0.15661950287728177}, {"Time"=3.3736821878559047, "delVelocity"=-0.14557389544094657}, {"Time"=3.376510638754095, "delVelocity"=-0.1349039128926497}, {"Time"=3.3793388982279513, "delVelocity"=-0.12462382571110331}, {"Time"=3.382167371726027, "delVelocity"=-0.11474483157163629}, {"Time"=3.384995909791781, "delVelocity"=-0.10527859350746338}, {"Time"=3.387824393364872, "delVelocity"=-0.09623496406471832}, {"Time"=3.3906527223172946, "delVelocity"=-0.0876220003959306}, {"Time"=3.393481108199337, "delVelocity"=-0.07944512204523047}, {"Time"=3.3963094377361482, "delVelocity"=-0.07170902084569752}, {"Time"=3.3991379663469496, "delVelocity"=-0.06441565722182996}, {"Time"=3.4019662626626093, "delVelocity"=-0.05756701186412039}, {"Time"=3.4047948122095746, "delVelocity"=-0.05116103741524025}, {"Time"=3.407623085681405, "delVelocity"=-0.04519630155219789}, {"Time"=3.410451795161922, "delVelocity"=-0.039666974292513424}, {"Time"=3.413280217362524, "delVelocity"=-0.03456841675003197}, {"Time"=3.416108504414759, "delVelocity"=-0.029892474275705516}, {"Time"=3.418937043764845, "delVelocity"=-0.025629080696520368}, {"Time"=3.4217654075327566, "delVelocity"=-0.021767816733099465}, {"Time"=3.424593812316918, "delVelocity"=-0.01829569099115136}, {"Time"=3.4274223098625938, "delVelocity"=-0.01519846382348422}, {"Time"=3.4302505771313307, "delVelocity"=-0.012460779733257099}, {"Time"=3.4330790782600054, "delVelocity"=-0.010065088700522806}, {"Time"=3.4359075150173846, "delVelocity"=-0.007993222069424322}, {"Time"=3.438736039883362, "delVelocity"=-0.006225341152230612}, {"Time"=3.4415643663019018, "delVelocity"=-0.004740678516154895}, {"Time"=3.4443929058556555, "delVelocity"=-0.003516972329440704}, {"Time"=3.4472213611723, "delVelocity"=-0.0025312911103164693}, {"Time"=3.450049696181311, "delVelocity"=-0.0017596062680016455}, {"Time"=3.452878186868382, "delVelocity"=-0.0011769853955369003}, {"Time"=3.4557066449019342, "delVelocity"=-0.0007578719156499103}, {"Time"=3.4585348683437767, "delVelocity"=-0.000476023381846824}, {"Time"=3.46136349809805, "delVelocity"=-0.00030459254236137046}, {"Time"=3.4641919499503446, "delVelocity"=-0.00021639700476427937}, {"Time"=3.4670203122318166, "delVelocity"=-0.00018386430809380627}, {"Time"=3.469848773705801, "delVelocity"=-0.00017921451859614912}]}, {[{"Time"=-0.19999971008368692, "delVelocity"=-0.00025347867963554984}, {"Time"=-0.19599955169521543, "delVelocity"=-0.0002468980755964031}, {"Time"=-0.19199972061079185, "delVelocity"=-0.00020087700608123035}, {"Time"=-0.18799993543103014, "delVelocity"=-7.613867600569091e-05}, {"Time"=-0.18399975382898923, "delVelocity"=0.0001663151231056191}, {"Time"=-0.1799997007453153, "delVelocity"=0.0005649747185511907}, {"Time"=-0.17599958135248003, "delVelocity"=0.0011577510798267377}, {"Time"=-0.1719996646246368, "delVelocity"=0.0019817201877715433}, {"Time"=-0.16799963988435399, "delVelocity"=0.00307315151916557}, {"Time"=-0.16399996028839184, "delVelocity"=0.004467050518843261}, {"Time"=-0.15999994591978378, "delVelocity"=0.006197614901672083}, {"Time"=-0.15599956522740924, "delVelocity"=0.008297587375635629}, {"Time"=-0.15199995070481703, "delVelocity"=0.010797493719106524}, {"Time"=-0.14799986563007528, "delVelocity"=0.013727660784965545}, {"Time"=-0.1439995266322304, "delVelocity"=0.017115952205084776}, {"Time"=-0.13999977230546354, "delVelocity"=0.020987694554953328}, {"Time"=-0.13599954645852697, "delVelocity"=0.025368076145006326}, {"Time"=-0.1319996384485409, "delVelocity"=0.030278440567770373}, {"Time"=-0.12799976226662602, "delVelocity"=0.03573915431578952}, {"Time"=-0.12399979238885099, "delVelocity"=0.04176831449516927}, {"Time"=-0.11999977801625923, "delVelocity"=0.04838154713329501}, {"Time"=-0.11599959711040041, "delVelocity"=0.055592467415114824}, {"Time"=-0.1119995663233781, "delVelocity"=0.06341151729769463}, {"Time"=-0.1079999864415866, "delVelocity"=0.07184657777366649}, {"Time"=-0.10399997974093139, "delVelocity"=0.0809056664821713}, {"Time"=-0.09999957195009002, "delVelocity"=0.09059263247208414}, {"Time"=-0.09599992718404889, "delVelocity"=0.10090581102189769}, {"Time"=-0.09199983345641843, "delVelocity"=0.11184701374850849}, {"Time"=-0.08799954749906208, "delVelocity"=0.12341197512527027}, {"Time"=-0.08399976840653432, "delVelocity"=0.13559242785161732}, {"Time"=-0.07999961390202075, "delVelocity"=0.14838241998902543}, {"Time"=-0.07599995197555989, "delVelocity"=0.1617681422140276}, {"Time"=-0.07199999465232532, "delVelocity"=0.17573882217630923}, {"Time"=-0.0679996101079472, "delVelocity"=0.19027940522055717}, {"Time"=-0.06399998128790332, "delVelocity"=0.2053676091977595}, {"Time"=-0.059999580272158445, "delVelocity"=0.22098911230699753}, {"Time"=-0.05599989537678559, "delVelocity"=0.2371159365506627}, {"Time"=-0.05199978214714182, "delVelocity"=0.25372845632419455}, {"Time"=-0.04799996317869244, "delVelocity"=0.2707976024886007}, {"Time"=-0.04399991978476187, "delVelocity"=0.2882976750379702}, {"Time"=-0.039999746775957065, "delVelocity"=0.3061987154462244}, {"Time"=-0.035999990487716675, "delVelocity"=0.3244670592488356}, {"Time"=-0.03199992598308618, "delVelocity"=0.34307336693474955}, {"Time"=-0.027999921938689717, "delVelocity"=0.36198199103931333}, {"Time"=-0.023999907204993128, "delVelocity"=0.38115810359991015}, {"Time"=-0.019999710005856947, "delVelocity"=0.40056633042810363}, {"Time"=-0.015999870245262362, "delVelocity"=0.420166911800768}, {"Time"=-0.011999536383572476, "delVelocity"=0.4399261331287043}, {"Time"=-0.007999854111300105, "delVelocity"=0.4597998209355175}, {"Time"=-0.003999539533107469, "delVelocity"=0.4797553765198303}, {"Time"=4.206370337300708e-07, "delVelocity"=0.499748601203626}, {"Time"=0.0040001928070261894, "delVelocity"=0.5197408826641763}, {"Time"=0.008000154213875661, "delVelocity"=0.5396946696982723}, {"Time"=0.01200029263836395, "delVelocity"=0.5595706106942616}, {"Time"=0.016000451168313144, "delVelocity"=0.5793289432235701}, {"Time"=0.020000149086689394, "delVelocity"=0.5989288072879799}, {"Time"=0.024000264861141582, "delVelocity"=0.6183366179276173}, {"Time"=0.02800004772495528, "delVelocity"=0.6375116040003344}, {"Time"=0.03200005186614291, "delVelocity"=0.6564202195902387}, {"Time"=0.036000074643543434, "delVelocity"=0.6750263248153721}, {"Time"=0.040000002099956106, "delVelocity"=0.6932954353050527}, {"Time"=0.0440003839006029, "delVelocity"=0.7111973753052635}, {"Time"=0.04800011545592462, "delVelocity"=0.7286960517545368}, {"Time"=0.05200034474566595, "delVelocity"=0.7457669090209483}, {"Time"=0.05600016904622125, "delVelocity"=0.7623781797682119}, {"Time"=0.0600002291765984, "delVelocity"=0.7785064595340736}, {"Time"=0.06400012142601703, "delVelocity"=0.7941259249085779}, {"Time"=0.06800009390001732, "delVelocity"=0.8092153829704625}, {"Time"=0.07200011094656215, "delVelocity"=0.82375458838516}, {"Time"=0.0760002094001565, "delVelocity"=0.8377257342943732}, {"Time"=0.08000015132865808, "delVelocity"=0.8511123348016744}, {"Time"=0.08400007704994006, "delVelocity"=0.8639015316859073}, {"Time"=0.08800000755570316, "delVelocity"=0.876082386572168}, {"Time"=0.09200003552494587, "delVelocity"=0.8876465507749618}, {"Time"=0.09600036516333599, "delVelocity"=0.8985883487130163}, {"Time"=0.1000003142478405, "delVelocity"=0.9089022193107297}, {"Time"=0.10400013989452307, "delVelocity"=0.9185877047979988}, {"Time"=0.10800042198737683, "delVelocity"=0.9276473706532675}, {"Time"=0.11200035326529989, "delVelocity"=0.9360830774495572}, {"Time"=0.11600034552580989, "delVelocity"=0.9439019343526269}, {"Time"=0.1200002911650988, "delVelocity"=0.9511123353456684}, {"Time"=0.1240004217682419, "delVelocity"=0.9577256757626124}, {"Time"=0.1280001980009166, "delVelocity"=0.9637544672404731}, {"Time"=0.13200031687336583, "delVelocity"=0.9692154344474546}, {"Time"=0.13600000342743665, "delVelocity"=0.9741254501770309}, {"Time"=0.1400002816864127, "delVelocity"=0.9785058264172676}, {"Time"=0.14400005880831768, "delVelocity"=0.9823775262207659}, {"Time"=0.1480000793127003, "delVelocity"=0.9857655037690816}, {"Time"=0.15200013456895942, "delVelocity"=0.9886956268999396}, {"Time"=0.1560000310376169, "delVelocity"=0.9911956759067333}, {"Time"=0.16000013543165031, "delVelocity"=0.993295471618897}, {"Time"=0.1640002914551009, "delVelocity"=0.9950260744006627}, {"Time"=0.16800007969886838, "delVelocity"=0.9964199805241443}, {"Time"=0.1720003672058504, "delVelocity"=0.9975114430156745}, {"Time"=0.17600026404218508, "delVelocity"=0.9983353648099454}, {"Time"=0.18000005915838904, "delVelocity"=0.9989280651738104}, {"Time"=0.1840003143581028, "delVelocity"=0.9993267249387076}, {"Time"=0.1880004350537107, "delVelocity"=0.9995691568364355}, {"Time"=0.19200001669955838, "delVelocity"=0.9996938788800452}, {"Time"=0.1960004297845222, "delVelocity"=0.9997398984442832}, {"Time"=0.20000036093943294, "delVelocity"=0.9997464747165504}, {"Time"=0.4414214913111456, "delVelocity"=1.0000742421887685}, {"Time"=0.44259297138594217, "delVelocity"=1.0000723152045665}, {"Time"=0.4437645032232444, "delVelocity"=1.0000588370679682}, {"Time"=0.4449361127671389, "delVelocity"=1.000022299583106}, {"Time"=0.44610776277175274, "delVelocity"=0.9999512839183818}, {"Time"=0.4472793422858625, "delVelocity"=0.9998345183600763}, {"Time"=0.44845091037450796, "delVelocity"=0.999660903264027}, {"Time"=0.4496224469605822, "delVelocity"=0.9994195713864208}, {"Time"=0.4507939451421718, "delVelocity"=0.999099925032463}, {"Time"=0.45196561733964014, "delVelocity"=0.9986915941259281}, {"Time"=0.45313709862923884, "delVelocity"=0.998184760894498}, {"Time"=0.4543087350264398, "delVelocity"=0.9975697207931465}, {"Time"=0.4554802630142199, "delVelocity"=0.9968374741517579}, {"Time"=0.45665192187030007, "delVelocity"=0.9959791977936256}, {"Time"=0.4578234273783297, "delVelocity"=0.9949869318226914}, {"Time"=0.45899508937649436, "delVelocity"=0.9938527694684679}, {"Time"=0.46016659440858865, "delVelocity"=0.9925699312024294}, {"Time"=0.4613381964469484, "delVelocity"=0.9911316540992428}, {"Time"=0.4625097692564046, "delVelocity"=0.9895321965731022}, {"Time"=0.4636812465114493, "delVelocity"=0.9877664288243592}, {"Time"=0.4648528237250482, "delVelocity"=0.9858294655894392}, {"Time"=0.4660245024438641, "delVelocity"=0.9837173447888735}, {"Time"=0.467196002511712, "delVelocity"=0.9814273645013661}, {"Time"=0.4683676149344291, "delVelocity"=0.978956449809889}, {"Time"=0.4695391933070697, "delVelocity"=0.9763030834312177}, {"Time"=0.4707106911089173, "delVelocity"=0.9734663100214884}, {"Time"=0.4718822733036999, "delVelocity"=0.9704453662466984}, {"Time"=0.4730538393858222, "delVelocity"=0.9672408582138691}, {"Time"=0.47422552679768126, "delVelocity"=0.9638534731049526}, {"Time"=0.47539705545723127, "delVelocity"=0.9602858374016313}, {"Time"=0.47656858974992344, "delVelocity"=0.9565400069611271}, {"Time"=0.47774019293172204, "delVelocity"=0.9526189869753567}, {"Time"=0.4789117431649517, "delVelocity"=0.9485270964514347}, {"Time"=0.48008330497801843, "delVelocity"=0.9442687089276309}, {"Time"=0.48125486758144903, "delVelocity"=0.9398491077391224}, {"Time"=0.48242654215769576, "delVelocity"=0.9352737342181119}, {"Time"=0.4835980037909976, "delVelocity"=0.9305503727284765}, {"Time"=0.4847696291261171, "delVelocity"=0.925684597795542}, {"Time"=0.4859412245624482, "delVelocity"=0.9206848324644334}, {"Time"=0.48711275030533785, "delVelocity"=0.9155594355506004}, {"Time"=0.4882843877939599, "delVelocity"=0.9103162763840393}, {"Time"=0.48945588431990333, "delVelocity"=0.9049656214983997}, {"Time"=0.4906275167504091, "delVelocity"=0.8995157663959553}, {"Time"=0.4917990739951855, "delVelocity"=0.8939776331062811}, {"Time"=0.49297065366887927, "delVelocity"=0.8883610639585815}, {"Time"=0.49414218370359725, "delVelocity"=0.8826770132145743}, {"Time"=0.4953137181154199, "delVelocity"=0.8769360957703451}, {"Time"=0.4964852885655416, "delVelocity"=0.8711492514198457}, {"Time"=0.4976569673483126, "delVelocity"=0.8653273952684726}, {"Time"=0.4988285264838186, "delVelocity"=0.8594830761848972}, {"Time"=0.5000000817405731, "delVelocity"=0.8536272261908296}, {"Time"=0.5011716196461153, "delVelocity"=0.8477714636736761}, {"Time"=0.5023431736722701, "delVelocity"=0.8419271721958766}, {"Time"=0.5035147631333795, "delVelocity"=0.8361057621622884}, {"Time"=0.5046864098031852, "delVelocity"=0.8303185444712468}, {"Time"=0.5058579934208131, "delVelocity"=0.8245773926237763}, {"Time"=0.5070294741753815, "delVelocity"=0.8188935890515184}, {"Time"=0.5082011203203837, "delVelocity"=0.8132767113373726}, {"Time"=0.5093726668714512, "delVelocity"=0.8077386420640345}, {"Time"=0.510544239436121, "delVelocity"=0.8022890776724554}, {"Time"=0.511715784258268, "delVelocity"=0.7969382152894287}, {"Time"=0.5128874356189028, "delVelocity"=0.7916950112841189}, {"Time"=0.5140589863433435, "delVelocity"=0.7865695256993416}, {"Time"=0.515230560515907, "delVelocity"=0.7815698733398846}, {"Time"=0.516402124305857, "delVelocity"=0.7767043726872893}, {"Time"=0.5175736521921331, "delVelocity"=0.7719807641039997}, {"Time"=0.5187451745853938, "delVelocity"=0.7674060001457914}, {"Time"=0.5199167610519144, "delVelocity"=0.7629863162594382}, {"Time"=0.5210883594783027, "delVelocity"=0.7587278074693479}, {"Time"=0.5222599659270958, "delVelocity"=0.7546357394654541}, {"Time"=0.523431567999114, "delVelocity"=0.7507147465864789}, {"Time"=0.52460303834387, "delVelocity"=0.7469691395640725}, {"Time"=0.5257746887215393, "delVelocity"=0.7434011569230766}, {"Time"=0.5269461800389071, "delVelocity"=0.7400143569252733}, {"Time"=0.5281178426131082, "delVelocity"=0.7368095955530389}, {"Time"=0.5292893402052617, "delVelocity"=0.7337888814804671}, {"Time"=0.5304608988095431, "delVelocity"=0.730951970524253}, {"Time"=0.5316325059984967, "delVelocity"=0.7282985555371251}, {"Time"=0.5328040454478186, "delVelocity"=0.72582780785388}, {"Time"=0.5339757035154437, "delVelocity"=0.7235375381499092}, {"Time"=0.5351472763768162, "delVelocity"=0.7214256312767511}, {"Time"=0.53631886470978, "delVelocity"=0.7194886652688208}, {"Time"=0.5374904347586501, "delVelocity"=0.7177227803401467}, {"Time"=0.5386619404308949, "delVelocity"=0.7161234383465288}, {"Time"=0.5398335273086352, "delVelocity"=0.714685197340128}, {"Time"=0.5410051671717525, "delVelocity"=0.7134022359361849}, {"Time"=0.5421766669878354, "delVelocity"=0.7122682524273996}, {"Time"=0.5433482557112554, "delVelocity"=0.7112759319467248}, {"Time"=0.5445198100855659, "delVelocity"=0.7104177461048269}, {"Time"=0.5456913675480461, "delVelocity"=0.709685490145307}, {"Time"=0.5468629436571404, "delVelocity"=0.7090704887029697}, {"Time"=0.5480346102538025, "delVelocity"=0.7085635870867552}, {"Time"=0.5492060748273954, "delVelocity"=0.7081553385796782}, {"Time"=0.5503777554626406, "delVelocity"=0.7078356502381788}, {"Time"=0.5515492835469495, "delVelocity"=0.707594332478564}, {"Time"=0.5527208220751906, "delVelocity"=0.7074207313160437}, {"Time"=0.5538924550767174, "delVelocity"=0.7073039687586938}, {"Time"=0.5550640457874608, "delVelocity"=0.7072329631833574}, {"Time"=0.5562355535573981, "delVelocity"=0.7071964316001176}, {"Time"=0.5574071858469414, "delVelocity"=0.7071829538072147}, {"Time"=0.5585786982270246, "delVelocity"=0.7071810275986217}, {"Time"=0.9242643843328034, "delVelocity"=0.7074652541686399}, {"Time"=0.9299215415096639, "delVelocity"=0.7074559489620098}, {"Time"=0.9355778619460791, "delVelocity"=0.7073908746677721}, {"Time"=0.9412351103002184, "delVelocity"=0.7072144502076033}, {"Time"=0.9468920964613852, "delVelocity"=0.7068715728985318}, {"Time"=0.9525486159623672, "delVelocity"=0.706307831457629}, {"Time"=0.9582055776981807, "delVelocity"=0.7054695494987538}, {"Time"=0.9638623863513119, "delVelocity"=0.7043042908862608}, {"Time"=0.9695192556755875, "delVelocity"=0.7027608055915503}, {"Time"=0.9751761766472402, "delVelocity"=0.7007893626292084}, {"Time"=0.9808331655452855, "delVelocity"=0.6983419078952219}, {"Time"=0.9864900148004712, "delVelocity"=0.6953723854180585}, {"Time"=0.9921465762271927, "delVelocity"=0.6918368428003372}, {"Time"=0.9978035839628779, "delVelocity"=0.6876929384798312}, {"Time"=1.0034606999240816, "delVelocity"=0.6829013683006023}, {"Time"=1.0091174011623711, "delVelocity"=0.6774257245755664}, {"Time"=1.0147740337876043, "delVelocity"=0.6712315605296624}, {"Time"=1.0204308963263573, "delVelocity"=0.6642871537161606}, {"Time"=1.0260875430322656, "delVelocity"=0.656564644593769}, {"Time"=1.0317447450907324, "delVelocity"=0.6480375739888212}, {"Time"=1.0374013564524076, "delVelocity"=0.6386855155747718}, {"Time"=1.0430586376918447, "delVelocity"=0.6284874629277561}, {"Time"=1.0487150631253201, "delVelocity"=0.6174306408050683}, {"Time"=1.0543722969597469, "delVelocity"=0.6054996328780202}, {"Time"=1.0600286135912673, "delVelocity"=0.5926893753529273}, {"Time"=1.0656859669093326, "delVelocity"=0.5789901631549979}, {"Time"=1.0713426284434175, "delVelocity"=0.5644043479804709}, {"Time"=1.076999193658818, "delVelocity"=0.548932332718922}, {"Time"=1.0826559896047643, "delVelocity"=0.5325784424052249}, {"Time"=1.088312876763294, "delVelocity"=0.5153517345267183}, {"Time"=1.093970040977261, "delVelocity"=0.4972637322345128}, {"Time"=1.0996270891013424, "delVelocity"=0.4783312261990491}, {"Time"=1.1052840039866023, "delVelocity"=0.4585732337326657}, {"Time"=1.1109406663472967, "delVelocity"=0.4380124173555534}, {"Time"=1.1165973998418814, "delVelocity"=0.4166729720074585}, {"Time"=1.1222544159869676, "delVelocity"=0.3945824337465645}, {"Time"=1.127911112467789, "delVelocity"=0.3717745271007525}, {"Time"=1.13356807899119, "delVelocity"=0.34828108693989124}, {"Time"=1.1392247416938168, "delVelocity"=0.3241414041187249}, {"Time"=1.1448818377574257, "delVelocity"=0.29939177172339954}, {"Time"=1.1505385374411603, "delVelocity"=0.2740776715831579}, {"Time"=1.1561952184196491, "delVelocity"=0.2482415663836362}, {"Time"=1.1618522272115093, "delVelocity"=0.22192798527854585}, {"Time"=1.1675088210159192, "delVelocity"=0.1951884232549317}, {"Time"=1.1731661004322718, "delVelocity"=0.1680673734717939}, {"Time"=1.1788228329607804, "delVelocity"=0.140621944849311}, {"Time"=1.1844796443155985, "delVelocity"=0.11290164609794162}, {"Time"=1.1901365103258799, "delVelocity"=0.08496017307735915}, {"Time"=1.195793302056504, "delVelocity"=0.05685262210848885}, {"Time"=1.2014499434300288, "delVelocity"=0.02863449319044542}, {"Time"=1.2071072601701265, "delVelocity"=0.0003572138048477669}, {"Time"=1.2127636414117435, "delVelocity"=-0.027915390136393103}, {"Time"=1.2184207205677626, "delVelocity"=-0.05613570547286373}, {"Time"=1.2240778879341696, "delVelocity"=-0.0842451174306823}, {"Time"=1.2297347952039583, "delVelocity"=-0.11218677986349312}, {"Time"=1.2353911037188137, "delVelocity"=-0.13990460668405158}, {"Time"=1.2410482721114244, "delVelocity"=-0.16735214147613953}, {"Time"=1.2467051623735093, "delVelocity"=-0.19447131484334512}, {"Time"=1.2523622238173289, "delVelocity"=-0.22121307163763304}, {"Time"=1.2580187388218105, "delVelocity"=-0.24752433992079848}, {"Time"=1.263675550725106, "delVelocity"=-0.27336104100793046}, {"Time"=1.2693327839558024, "delVelocity"=-0.29867749429031765}, {"Time"=1.2749892892635577, "delVelocity"=-0.3234245086185723}, {"Time"=1.2806464197553922, "delVelocity"=-0.34756615803350854}, {"Time"=1.2863030240186304, "delVelocity"=-0.3710580565051329}, {"Time"=1.2919602723344672, "delVelocity"=-0.3938681367003154}, {"Time"=1.297616528864611, "delVelocity"=-0.4159556689601369}, {"Time"=1.3032735322811533, "delVelocity"=-0.4372961238410862}, {"Time"=1.3089303589311432, "delVelocity"=-0.45785749802498077}, {"Time"=1.3145874415976353, "delVelocity"=-0.4776160120445023}, {"Time"=1.3202439225437799, "delVelocity"=-0.49654658354447645}, {"Time"=1.3259010657286179, "delVelocity"=-0.5146345256915887}, {"Time"=1.33155785866155, "delVelocity"=-0.5318609626805202}, {"Time"=1.3372150380138068, "delVelocity"=-0.5482159551784207}, {"Time"=1.3428712965693161, "delVelocity"=-0.563687119429789}, {"Time"=1.3485286000635486, "delVelocity"=-0.5782745512767336}, {"Time"=1.3541855979258655, "delVelocity"=-0.5919728416299201}, {"Time"=1.3598424176086192, "delVelocity"=-0.6047841660899749}, {"Time"=1.365499326431115, "delVelocity"=-0.6167144028938447}, {"Time"=1.371155774914977, "delVelocity"=-0.6277712086081537}, {"Time"=1.376812934662422, "delVelocity"=-0.6379689891509921}, {"Time"=1.3824693199948028, "delVelocity"=-0.6473206474930489}, {"Time"=1.3881263804328017, "delVelocity"=-0.6558475054131294}, {"Time"=1.3937836314703784, "delVelocity"=-0.6635708082245788}, {"Time"=1.3994402025755186, "delVelocity"=-0.6705148055019887}, {"Time"=1.4050967144670052, "delVelocity"=-0.67670881442554}, {"Time"=1.4107541949346079, "delVelocity"=-0.68218515012525}, {"Time"=1.4164107073228933, "delVelocity"=-0.6869761388864155}, {"Time"=1.4220677524359233, "delVelocity"=-0.6911200361835448}, {"Time"=1.4277242140185793, "delVelocity"=-0.694655487385275}, {"Time"=1.4333815111780939, "delVelocity"=-0.6976252016907452}, {"Time"=1.43903800462069, "delVelocity"=-0.7000724038643951}, {"Time"=1.4446951947442999, "delVelocity"=-0.7020439155647842}, {"Time"=1.450351948312078, "delVelocity"=-0.7035873412023061}, {"Time"=1.4560090025978079, "delVelocity"=-0.7047526220630205}, {"Time"=1.4616654599202634, "delVelocity"=-0.7055908114315721}, {"Time"=1.4673224279161987, "delVelocity"=-0.7061545847737003}, {"Time"=1.4729793714749515, "delVelocity"=-0.7064974422305579}, {"Time"=1.4786361713695508, "delVelocity"=-0.7066738460135511}, {"Time"=1.4842927414440474, "delVelocity"=-0.7067389210470298}, {"Time"=1.4899497767315795, "delVelocity"=-0.7067482248576791}]}]
  out "yAccel":T2(array[cluster])=[{"A"=5.0, "B"=7.853981633974483, "Start"=-0.2, "End"=0.2, "Center"=0.0, "Velocity"=0.0, "Position"=1.0}, {"A"=-5.0, "B"=26.815170613344876, "Start"=0.4414213562373095, "End"=0.5585786437626905, "Center"=0.5, "Velocity"=1.0, "Position"=0.7071067811865475}, {"A"=-5.0, "B"=5.553603672697958, "Start"=0.9242640687119285, "End"=1.4899494936611664, "Center"=1.2071067811865475, "Velocity"=0.7071067811865475, "Position"=-0.7071067811865475}, {"A"=5.0, "B"=5.553603672697958, "Start"=2.3384776310850235, "End"=2.9041630560342613, "Center"=2.6213203435596424, "Velocity"=-0.7071067811865475, "Position"=0.7071067811865475}, {"A"=-5.0, "B"=4.60075592255305, "Start"=2.9870057685088804, "End"=3.6698484809834993, "Center"=3.32842712474619, "Velocity"=0.7071067811865475, "Position"=-1.0}]
  out "xAccel":T2(array[cluster])=[{"A"=5.0, "B"=11.107207345395915, "Start"=0.3585786437626905, "End"=0.6414213562373094, "Center"=0.5, "Velocity"=0.0, "Position"=0.7071067811865475}, {"A"=-5.0, "B"=5.553603672697958, "Start"=1.631370849898476, "End"=2.197056274847714, "Center"=1.914213562373095, "Velocity"=0.7071067811865475, "Position"=-0.7071067811865475}, {"A"=5.0, "B"=11.107207345395915, "Start"=3.18700576850888, "End"=3.4698484809834995, "Center"=3.32842712474619, "Velocity"=-0.7071067811865475, "Position"=0.0}]
  out "Yvel":cluster{dbl, dbl, dbl}[](array[cluster])=[{0.0, 1.0, 0.5}, {0.5, 0.7071067811865475, 1.0}, {1.2071067811865475, -0.7071067811865475, 0.5}, {1.914213562373095, -0.7071067811865475, 0.0}, {2.6213203435596424, 0.7071067811865475, 0.5}, {3.32842712474619, -1.0, 0.0}, {3.82842712474619, -1.0, 0.5}]
  out "Xvel":cluster{dbl, dbl, dbl}[](array[cluster])=[{0.0, 0.0, 0.0}, {0.5, 0.7071067811865475, 0.5}, {1.2071067811865475, 0.7071067811865475, 1.0}, {1.914213562373095, -0.7071067811865475, 0.5}, {2.6213203435596424, -0.7071067811865475, 0.0}, {3.32842712474619, 0.0, 0.0}, {3.82842712474619, 0.0, 0.0}]
  out "Accel":cluster{cluster{"Time":dbl, "Velocity":dbl}[]}[](graph)=[{[{"Time"=0.3585786539181065, "Velocity"=1.3064499120456236e-13}, {"Time"=0.36140731109565516, "Velocity"=0.0049340316337055014}, {"Time"=0.3642357307917301, "Velocity"=0.01971489639868962}, {"Time"=0.3670642068784426, "Velocity"=0.04428484816558497}, {"Time"=0.3698926688739745, "Velocity"=0.07854652593049968}, {"Time"=0.37272085534132177, "Velocity"=0.12236008069645293}, {"Time"=0.37554943458046675, "Velocity"=0.17556352711837556}, {"Time"=0.37837782561733807, "Velocity"=0.2379369978974781}, {"Time"=0.3812060928086513, "Velocity"=0.3092342561591022}, {"Time"=0.3840346631145527, "Velocity"=0.3891855079872978}, {"Time"=0.3868632343372613, "Velocity"=0.4774680528379116}, {"Time"=0.38969151605783653, "Velocity"=0.5737231713774339}, {"Time"=0.3925199825155379, "Velocity"=0.677586665886694}, {"Time"=0.3953483936939714, "Velocity"=0.7886403548293002}, {"Time"=0.39817695281408544, "Velocity"=0.9064542525346031}, {"Time"=0.4010052846136086, "Velocity"=1.0305475202151184}, {"Time"=0.4038334793365938, "Velocity"=1.1604332267682187}, {"Time"=0.40666210983592205, "Velocity"=1.2956259303563127}, {"Time"=0.40949054770928306, "Velocity"=1.4355627516245575}, {"Time"=0.41231892145882515, "Velocity"=1.5796971409639606}, {"Time"=0.41514750834379105, "Velocity"=1.7274746653677187}, {"Time"=0.4179758305988945, "Velocity"=1.8782871036522448}, {"Time"=0.4208041109913757, "Velocity"=2.0315506929652867}, {"Time"=0.42363258179681645, "Velocity"=2.1866733372099993}, {"Time"=0.4264610538905579, "Velocity"=2.3430326481576373}, {"Time"=0.42928951171659996, "Velocity"=2.5000106648132463}, {"Time"=0.4321177938793383, "Velocity"=2.656978902987783}, {"Time"=0.43494643070376915, "Velocity"=2.8133472218555173}, {"Time"=0.43777478007766585, "Velocity"=2.968463038077345}, {"Time"=0.44060328955956823, "Velocity"=3.121738758836332}, {"Time"=0.4434316661934197, "Velocity"=3.272553601321946}, {"Time"=0.4462599440832893, "Velocity"=3.420314537946749}, {"Time"=0.4490885886953773, "Velocity"=3.5644622248638274}, {"Time"=0.4519170662885518, "Velocity"=3.704400191883474}, {"Time"=0.4547453849155592, "Velocity"=3.8395773183162207}, {"Time"=0.4575739111245775, "Velocity"=3.9694774773920436}, {"Time"=0.4604021855054836, "Velocity"=4.0935670983890295}, {"Time"=0.4632306519590422, "Velocity"=4.211376093345904}, {"Time"=0.46605895683881216, "Velocity"=4.322424738837032}, {"Time"=0.4688875417410551, "Velocity"=4.426291641171033}, {"Time"=0.4717159852119831, "Velocity"=4.522550886288434}, {"Time"=0.4745444223356806, "Velocity"=4.610827766461567}, {"Time"=0.4773728319436485, "Velocity"=4.690773379257046}, {"Time"=0.48020113490224603, "Velocity"=4.762070596167143}, {"Time"=0.48302967462562646, "Velocity"=4.824446078395532}, {"Time"=0.48585817794251845, "Velocity"=4.8776466795190565}, {"Time"=0.4886864284978635, "Velocity"=4.921459799767104}, {"Time"=0.49151488324395665, "Velocity"=4.955719842636414}, {"Time"=0.4943432951580636, "Velocity"=4.980287794449829}, {"Time"=0.49717157354251873, "Velocity"=4.9950668237042315}, {"Time"=0.5000003039005825, "Velocity"=4.9999999999430305}, {"Time"=0.5028285215961745, "Velocity"=4.995066491937139}, {"Time"=0.5056570599371091, "Velocity"=4.9802853227938755}, {"Time"=0.5084853935880203, "Velocity"=4.955716961816788}, {"Time"=0.5113140271325607, "Velocity"=4.921453506892027}, {"Time"=0.5141421725071926, "Velocity"=4.877640665305854}, {"Time"=0.5169707086497233, "Velocity"=4.824438242666381}, {"Time"=0.5197990029218125, "Velocity"=4.762067337175239}, {"Time"=0.522627645640868, "Velocity"=4.690760601637483}, {"Time"=0.5254558585788796, "Velocity"=4.6108194071286865}, {"Time"=0.5282844167278493, "Velocity"=4.522537765683651}, {"Time"=0.5311128114392702, "Velocity"=4.426279138608812}, {"Time"=0.5339411977017692, "Velocity"=4.322418863663652}, {"Time"=0.5367697787927276, "Velocity"=4.211358654776027}, {"Time"=0.539598270019943, "Velocity"=4.093547605864477}, {"Time"=0.5424265788585229, "Velocity"=3.969455462675649}, {"Time"=0.5452551677080153, "Velocity"=3.8395514054308446}, {"Time"=0.5480833252623692, "Velocity"=3.704381136463005}, {"Time"=0.5509120002803135, "Velocity"=3.5644326285319}, {"Time"=0.5537402466559421, "Velocity"=3.4203046889138577}, {"Time"=0.5565687529512425, "Velocity"=3.272531462977887}, {"Time"=0.5593971983085523, "Velocity"=3.1217125157939076}, {"Time"=0.5622257013470414, "Velocity"=2.968436775226552}, {"Time"=0.5650540471136181, "Velocity"=2.8133208950186264}, {"Time"=0.5678824150643235, "Velocity"=2.6569673219819907}, {"Time"=0.5707108477885655, "Velocity"=2.499990699321794}, {"Time"=0.5735394142333143, "Velocity"=2.3430067017171288}, {"Time"=0.5763677396701484, "Velocity"=2.186655624987825}, {"Time"=0.579196171936455, "Velocity"=2.0315352585947952}, {"Time"=0.5820244417111652, "Velocity"=1.8782724557417694}, {"Time"=0.5848528155359576, "Velocity"=1.727457558696861}, {"Time"=0.5876815668613797, "Velocity"=1.5796719260308365}, {"Time"=0.5905096733818155, "Velocity"=1.4355516416722565}, {"Time"=0.593338196086523, "Velocity"=1.295611042141539}, {"Time"=0.5961666624872919, "Velocity"=1.1604265765637671}, {"Time"=0.5989951160040351, "Velocity"=1.0305295206155138}, {"Time"=0.6018236883773812, "Velocity"=0.9064268151439998}, {"Time"=0.6046519490296856, "Velocity"=0.7886264799869956}, {"Time"=0.6074802321291861, "Velocity"=0.6775785057102515}, {"Time"=0.6103086871531369, "Velocity"=0.5737159776941383}, {"Time"=0.6131372908708361, "Velocity"=0.4774509083006246}, {"Time"=0.6159658038737286, "Velocity"=0.38917161151874513}, {"Time"=0.6187941476790058, "Velocity"=0.30922782200862176}, {"Time"=0.6216223788804354, "Velocity"=0.23793216230263123}, {"Time"=0.6244508586079508, "Velocity"=0.17555753309346528}, {"Time"=0.6272793672652286, "Velocity"=0.1223562604248374}, {"Time"=0.6301077028527967, "Velocity"=0.07854139185915301}, {"Time"=0.6329361356658376, "Velocity"=0.04428128345999199}, {"Time"=0.6357648050406953, "Velocity"=0.019711166751556295}, {"Time"=0.6385931085896726, "Velocity"=0.004932568115766509}, {"Time"=0.6414214564562928, "Velocity"=5.663743054542054e-12}, {"Time"=1.6313709389722086, "Velocity"=-2.05700306145328e-11}, {"Time"=1.6370282817767798, "Velocity"=-0.004933394551697377}, {"Time"=1.6426852164065096, "Velocity"=-0.019713958013341998}, {"Time"=1.6483420602555467, "Velocity"=-0.044282884232342445}, {"Time"=1.6539986065707935, "Velocity"=-0.0785413148532954}, {"Time"=1.6596555285100723, "Velocity"=-0.12235832085132031}, {"Time"=1.6653120260845347, "Velocity"=-0.17555468004132713}, {"Time"=1.6709691479513475, "Velocity"=-0.23793078861467062}, {"Time"=1.676626210753658, "Velocity"=-0.30923430626988446}, {"Time"=1.6822830849701813, "Velocity"=-0.3891816076300143}, {"Time"=1.687939861008537, "Velocity"=-0.4774578021843385}, {"Time"=1.6935967721537473, "Velocity"=-0.5737182184701481}, {"Time"=1.6992535618174427, "Velocity"=-0.6775786334964428}, {"Time"=1.7049101385312582, "Velocity"=-0.7886268392141059}, {"Time"=1.7105673666365064, "Velocity"=-0.9064423281475641}, {"Time"=1.7162237653047285, "Velocity"=-1.030529059805671}, {"Time"=1.7218807229541682, "Velocity"=-1.1604272942861342}, {"Time"=1.7275375237543296, "Velocity"=-1.2956085874163001}, {"Time"=1.733194444417825, "Velocity"=-1.43554598557842}, {"Time"=1.7388511259374029, "Velocity"=-1.5796782223146013}, {"Time"=1.7445079508551682, "Velocity"=-1.727446114337209}, {"Time"=1.7501651561700786, "Velocity"=-1.8782731233671692}, {"Time"=1.7558217908902145, "Velocity"=-2.0315385454475057}, {"Time"=1.7614787580989848, "Velocity"=-2.1866617873866834}, {"Time"=1.767135947698282, "Velocity"=-2.343027844775897}, {"Time"=1.7727925205886734, "Velocity"=-2.499996348263935}, {"Time"=1.7784496447984022, "Velocity"=-2.656980145001215}, {"Time"=1.784106337495474, "Velocity"=-2.813332465872235}, {"Time"=1.7897629599964713, "Velocity"=-2.968446362427656}, {"Time"=1.795419991649167, "Velocity"=-3.121722670814489}, {"Time"=1.8010766261793898, "Velocity"=-3.2725346821260892}, {"Time"=1.8067339869267998, "Velocity"=-3.4203168379103897}, {"Time"=1.8123907905214702, "Velocity"=-3.564452274362697}, {"Time"=1.8180472737360638, "Velocity"=-3.7043790827974803}, {"Time"=1.8237045187665355, "Velocity"=-3.8395712409927047}, {"Time"=1.8293608161022459, "Velocity"=-3.969454702909954}, {"Time"=1.835018222910025, "Velocity"=-4.093563777131078}, {"Time"=1.8406749007109258, "Velocity"=-4.211367797619743}, {"Time"=1.8463315025365392, "Velocity"=-4.322416807479287}, {"Time"=1.8519887578682013, "Velocity"=-4.426285778669941}, {"Time"=1.857645415280835, "Velocity"=-4.5225417423543375}, {"Time"=1.863302429809249, "Velocity"=-4.610821525627349}, {"Time"=1.8689589505381832, "Velocity"=-4.690763782063026}, {"Time"=1.8746160614660987, "Velocity"=-4.762068090831172}, {"Time"=1.8802728803168463, "Velocity"=-4.824441253702339}, {"Time"=1.8859293786998357, "Velocity"=-4.87763827268736}, {"Time"=1.891586246485062, "Velocity"=-4.921455569735294}, {"Time"=1.897243038606047, "Velocity"=-4.9557160473581146}, {"Time"=1.9029001401610677, "Velocity"=-4.980286224260394}, {"Time"=1.9085573116801937, "Velocity"=-4.995067109794932}, {"Time"=1.9142136891534374, "Velocity"=-4.999999999985098}, {"Time"=1.9198710239034444, "Velocity"=-4.995066524681679}, {"Time"=1.9255277598812142, "Velocity"=-4.980286572141937}, {"Time"=1.9311845207804696, "Velocity"=-4.9557183399856966}, {"Time"=1.9368410274551104, "Velocity"=-4.921460583627283}, {"Time"=1.9424979175158914, "Velocity"=-4.877644311712433}, {"Time"=1.9481552889708231, "Velocity"=-4.824439523224635}, {"Time"=1.953811592279, "Velocity"=-4.762072184598966}, {"Time"=1.9594690660596115, "Velocity"=-4.690763560027577}, {"Time"=1.9651255485412915, "Velocity"=-4.610821847745683}, {"Time"=1.9707825825585772, "Velocity"=-4.522541777618684}, {"Time"=1.9764390196790906, "Velocity"=-4.426289716069483}, {"Time"=1.9820958981581804, "Velocity"=-4.3224281993777085}, {"Time"=1.9877530377406014, "Velocity"=-4.211369043484462}, {"Time"=1.9934097229876202, "Velocity"=-4.093564934682716}, {"Time"=1.999066945741638, "Velocity"=-3.969460053050553}, {"Time"=2.0047234227059696, "Velocity"=-3.8395726131862085}, {"Time"=2.010380087442325, "Velocity"=-3.704394627425888}, {"Time"=2.016037078197146, "Velocity"=-3.5644555728371294}, {"Time"=2.0216939876419815, "Velocity"=-3.4203174944942765}, {"Time"=2.0273506595959043, "Velocity"=-3.272553544050992}, {"Time"=2.033007989055367, "Velocity"=-3.121723189778432}, {"Time"=2.0386643720067625, "Velocity"=-2.968464582819272}, {"Time"=2.0443217298911254, "Velocity"=-2.8133306094345656}, {"Time"=2.04997821198491, "Velocity"=-2.6569841139970967}, {"Time"=2.055634964753559, "Velocity"=-2.5000106392911285}, {"Time"=2.0612919001257297, "Velocity"=-2.343032062064146}, {"Time"=2.0669492981152833, "Velocity"=-2.1866602387368608}, {"Time"=2.072605554961524, "Velocity"=-2.0315563881090606}, {"Time"=2.0782629610608425, "Velocity"=-1.8782699703681704}, {"Time"=2.08391953438395, "Velocity"=-1.7274597086263335}, {"Time"=2.089576586863454, "Velocity"=-1.5796856372285875}, {"Time"=2.0952334244867075, "Velocity"=-1.4355492793827267}, {"Time"=2.100890129859104, "Velocity"=-1.295617016138658}, {"Time"=2.106547045189576, "Velocity"=-1.160432730224122}, {"Time"=2.1122039402292123, "Velocity"=-1.030535674916126}, {"Time"=2.1178604687787836, "Velocity"=-0.9064458495467985}, {"Time"=2.1235173794696283, "Velocity"=-0.788636595844999}, {"Time"=2.1291744509901696, "Velocity"=-0.6775783900427088}, {"Time"=2.134830881736091, "Velocity"=-0.5737243446411354}, {"Time"=2.140487756116038, "Velocity"=-0.4774640513563506}, {"Time"=2.146145015007327, "Velocity"=-0.3891801200785638}, {"Time"=2.151801554995862, "Velocity"=-0.3092374399317057}, {"Time"=2.1574584285988165, "Velocity"=-0.23793579509158463}, {"Time"=2.1631155242830973, "Velocity"=-0.17555927620104034}, {"Time"=2.1687721832366433, "Velocity"=-0.12236079430060422}, {"Time"=2.1744294685497514, "Velocity"=-0.07854079610231214}, {"Time"=2.1800860456828968, "Velocity"=-0.04428233300804034}, {"Time"=2.185743085377008, "Velocity"=-0.019712907724584734}, {"Time"=2.1913998992840336, "Velocity"=-0.004933078857937823}, {"Time"=2.1970563810962314, "Velocity"=-1.5273488367710927e-11}, {"Time"=3.1870060479132465, "Velocity"=1.0295951656901158e-10}, {"Time"=3.1898342454717667, "Velocity"=0.0049338027771435675}, {"Time"=3.192662685302619, "Velocity"=0.01971457975930896}, {"Time"=3.1954913108213567, "Velocity"=0.04428592988126721}, {"Time"=3.1983194823650973, "Velocity"=0.0785439499590373}, {"Time"=3.2011480219442108, "Velocity"=0.12236293989693467}, {"Time"=3.203976578187884, "Velocity"=0.1755664631040197}, {"Time"=3.206804864653635, "Velocity"=0.2379379209627888}, {"Time"=3.2096332640061265, "Velocity"=0.3092388365167493}, {"Time"=3.2124616323706507, "Velocity"=0.38918459311438536}, {"Time"=3.2152900788124303, "Velocity"=0.4774629759620106}, {"Time"=3.2181185852393797, "Velocity"=0.5737256204180676}, {"Time"=3.220947081278704, "Velocity"=0.6775904205927669}, {"Time"=3.223775590960444, "Velocity"=0.7886483410203865}, {"Time"=3.226604029368186, "Velocity"=0.906457528402615}, {"Time"=3.229432511192091, "Velocity"=1.030557700352381}, {"Time"=3.2322606966840968, "Velocity"=1.1604434183447923}, {"Time"=3.2350892011195653, "Velocity"=1.2956303728344774}, {"Time"=3.2379175263860533, "Velocity"=1.4355616801191275}, {"Time"=3.2407459278022506, "Velocity"=1.5796974685141905}, {"Time"=3.2435743709266927, "Velocity"=1.7274674072706475}, {"Time"=3.2464028937659486, "Velocity"=1.8782905014930729}, {"Time"=3.2492314737397603, "Velocity"=2.0315704817595086}, {"Time"=3.2520596094987266, "Velocity"=2.1866748635336384}, {"Time"=3.254888337065098, "Velocity"=2.343048343523004}, {"Time"=3.2577164493945463, "Velocity"=2.5000072036934915}, {"Time"=3.260544904978059, "Velocity"=2.6569850607942924}, {"Time"=3.26337351450344, "Velocity"=2.813351839055695}, {"Time"=3.2662018882206443, "Velocity"=2.9684689375239586}, {"Time"=3.2690302397129716, "Velocity"=3.121736077528286}, {"Time"=3.271858810452424, "Velocity"=3.272561220765227}, {"Time"=3.2746871016510424, "Velocity"=3.420322674120906}, {"Time"=3.2775155542714263, "Velocity"=3.5644604950475633}, {"Time"=3.2803438853865963, "Velocity"=3.7043913880262815}, {"Time"=3.283172577802294, "Velocity"=3.8395863628554205}, {"Time"=3.2860009988928733, "Velocity"=3.96948142076301}, {"Time"=3.2888292025801555, "Velocity"=4.0935678290332405}, {"Time"=3.2916577959736606, "Velocity"=4.211381923603854}, {"Time"=3.294486165196214, "Velocity"=4.3224326599319065}, {"Time"=3.2973147419065647, "Velocity"=4.426298726965357}, {"Time"=3.3001430501176015, "Velocity"=4.522553005000786}, {"Time"=3.3029713594790264, "Velocity"=4.610825896007822}, {"Time"=3.3057997085757598, "Velocity"=4.690770078612631}, {"Time"=3.3086282731289107, "Velocity"=4.762073864657787}, {"Time"=3.3114568801153026, "Velocity"=4.824450279382761}, {"Time"=3.314285247666322, "Velocity"=4.8776478760610535}, {"Time"=3.317113460494852, "Velocity"=4.921460241679657}, {"Time"=3.31994201821709, "Velocity"=4.955721247184877}, {"Time"=3.3227703109610096, "Velocity"=4.98028790444336}, {"Time"=3.325598955394788, "Velocity"=4.995068155185091}, {"Time"=3.3284273788279397, "Velocity"=4.999999999911475}, {"Time"=3.3312557348684333, "Velocity"=4.995065748174875}, {"Time"=3.334084180211739, "Velocity"=4.980284485581901}, {"Time"=3.336912519985483, "Velocity"=4.955715646445476}, {"Time"=3.339740957077332, "Velocity"=4.921454474466035}, {"Time"=3.3425695055356752, "Velocity"=4.877634949932064}, {"Time"=3.345397798516264, "Velocity"=4.824436405399207}, {"Time"=3.348226161536805, "Velocity"=4.762063586534025}, {"Time"=3.3510547853629995, "Velocity"=4.69075686337034}, {"Time"=3.3538832913057233, "Velocity"=4.610806530071291}, {"Time"=3.356711404873941, "Velocity"=4.522538152635537}, {"Time"=3.3595399011777736, "Velocity"=4.426275961852315}, {"Time"=3.3623684919508743, "Velocity"=4.322407677128236}, {"Time"=3.365196989354992, "Velocity"=4.211350130308858}, {"Time"=3.3680253602013126, "Velocity"=4.093543746867211}, {"Time"=3.37085380375171, "Velocity"=3.9694453582694145}, {"Time"=3.3736821904673313, "Velocity"=3.8395503382271174}, {"Time"=3.376510575544337, "Velocity"=3.704368956063038}, {"Time"=3.3793389541262036, "Velocity"=3.5644349478062862}, {"Time"=3.382167301528867, "Velocity"=3.420301855486132}, {"Time"=3.3849959552185953, "Velocity"=3.272520779615571}, {"Time"=3.3878242330712953, "Velocity"=3.1217106458592654}, {"Time"=3.3906525359645023, "Velocity"=2.9684457972393226}, {"Time"=3.393481003787624, "Velocity"=2.8133232822006473}, {"Time"=3.39630971133789, "Velocity"=2.65695090058365}, {"Time"=3.3991378836616883, "Velocity"=2.499988707070791}, {"Time"=3.401966565931198, "Velocity"=2.3429982936468585}, {"Time"=3.40479482134524, "Velocity"=2.18665112484719}, {"Time"=3.407623243021488, "Velocity"=2.0315313807440107}, {"Time"=3.4104515208080355, "Velocity"=1.87826820102303}, {"Time"=3.413280220885957, "Velocity"=1.7274361489890873}, {"Time"=3.41610838513316, "Velocity"=1.5796813097480884}, {"Time"=3.418937062665855, "Velocity"=1.4355320799922966}, {"Time"=3.4217654402904434, "Velocity"=1.295599157599364}, {"Time"=3.4245938304906525, "Velocity"=1.1604186988057235}, {"Time"=3.4274223156270405, "Velocity"=1.030520551672633}, {"Time"=3.4302506894641223, "Velocity"=0.9064267686412566}, {"Time"=3.433079034797023, "Velocity"=0.788623007793185}, {"Time"=3.4359073642324387, "Velocity"=0.677573483544283}, {"Time"=3.438735804071094, "Velocity"=0.5737118388077107}, {"Time"=3.4415642218030187, "Velocity"=0.4774531628879406}, {"Time"=3.444392723790257, "Velocity"=0.3891739945976159}, {"Time"=3.4472212731111203, "Velocity"=0.3092244661476888}, {"Time"=3.4500497619347352, "Velocity"=0.23792310465042021}, {"Time"=3.4528781482091495, "Velocity"=0.17555161250344603}, {"Time"=3.455706613162803, "Velocity"=0.12235204051092692}, {"Time"=3.4585349141655324, "Velocity"=0.0785384734056483}, {"Time"=3.4613634374995264, "Velocity"=0.04427814252922244}, {"Time"=3.464191679311487, "Velocity"=0.01971204185476132}, {"Time"=3.467020269738526, "Velocity"=0.004932006218463123}, {"Time"=3.469848546439775, "Velocity"=2.1295770158577255e-11}]}, {[{"Time"=-0.1999995259633287, "Velocity"=6.660776896146807e-11}, {"Time"=-0.19599992610834677, "Velocity"=0.004933338607754894}, {"Time"=-0.1919997681269363, "Velocity"=0.019714343927452537}, {"Time"=-0.1879999837960189, "Velocity"=0.04428192794327498}, {"Time"=-0.1839997238460617, "Velocity"=0.07854471038261848}, {"Time"=-0.17999985299987104, "Velocity"=0.12236039132724731}, {"Time"=-0.1759999899995893, "Velocity"=0.17555881127366782}, {"Time"=-0.17199959843555093, "Velocity"=0.23793894913440472}, {"Time"=-0.16799968751027647, "Velocity"=0.30923906360765735}, {"Time"=-0.1639998102194453, "Velocity"=0.38918401876781555}, {"Time"=-0.15999957008121524, "Velocity"=0.47746726549481305}, {"Time"=-0.15599984475619627, "Velocity"=0.573720597079356}, {"Time"=-0.1519998088763115, "Velocity"=0.6775833788339134}, {"Time"=-0.14799967696562544, "Velocity"=0.7886412851057385}, {"Time"=-0.14399960906382744, "Velocity"=0.9064516515386111}, {"Time"=-0.13999975526276712, "Velocity"=1.0305444373023989}, {"Time"=-0.13599992553550386, "Velocity"=1.160435271397883}, {"Time"=-0.13199989559332662, "Velocity"=1.2956191959447714}, {"Time"=-0.12799978957733887, "Velocity"=1.4355590359696915}, {"Time"=-0.12399954219524378, "Velocity"=1.579705122788552}, {"Time"=-0.11999978348071712, "Velocity"=1.7274653917416476}, {"Time"=-0.11599963110954292, "Velocity"=1.8782891076542803}, {"Time"=-0.11199969698166555, "Velocity"=2.0315582009269963}, {"Time"=-0.10799966698364727, "Velocity"=2.186679694400209}, {"Time"=-0.1039996477785454, "Velocity"=2.3430373156324764}, {"Time"=-0.09999976657755182, "Velocity"=2.500008983465774}, {"Time"=-0.09599983363219963, "Velocity"=2.6569826438338895}, {"Time"=-0.09199999418256315, "Velocity"=2.813333143515508}, {"Time"=-0.08799963052307017, "Velocity"=2.9684673805837614}, {"Time"=-0.08399981742947535, "Velocity"=3.1217315132928682}, {"Time"=-0.07999993190170934, "Velocity"=3.272544890021001}, {"Time"=-0.07599994169894399, "Velocity"=3.4203133810911126}, {"Time"=-0.07199991158179106, "Velocity"=3.5644512514013753}, {"Time"=-0.06799957255227443, "Velocity"=3.704398785710548}, {"Time"=-0.06399968780101505, "Velocity"=3.839577240019463}, {"Time"=-0.05999982778626195, "Velocity"=3.9694685131244074}, {"Time"=-0.05599978113691681, "Velocity"=4.093566517750869}, {"Time"=-0.051999699334965004, "Velocity"=4.211376302426815}, {"Time"=-0.04799997263022988, "Velocity"=4.322422244175563}, {"Time"=-0.04399990007940245, "Velocity"=4.426285556778941}, {"Time"=-0.03999974807045133, "Velocity"=4.522548257999745}, {"Time"=-0.03599970539484101, "Velocity"=4.610825977473423}, {"Time"=-0.03199963124895329, "Velocity"=4.690773648048182}, {"Time"=-0.02799993046373069, "Velocity"=4.7620687720135875}, {"Time"=-0.023999819356509255, "Velocity"=4.82444380996392}, {"Time"=-0.019999885810602972, "Velocity"=4.877642665119586}, {"Time"=-0.015999642032533137, "Velocity"=4.921461391422147}, {"Time"=-0.011999651760680845, "Velocity"=4.955720685170617}, {"Time"=-0.007999805879442913, "Velocity"=4.980287706867074}, {"Time"=-0.003999779930066721, "Velocity"=4.995067363239748}, {"Time"=3.082748587200181e-07, "Velocity"=4.999999999970689}, {"Time"=0.004000234939050095, "Velocity"=4.99506624128645}, {"Time"=0.008000444434326806, "Velocity"=4.980284563962754}, {"Time"=0.012000373173285197, "Velocity"=4.955715376688249}, {"Time"=0.016000136941335924, "Velocity"=4.921456558160642}, {"Time"=0.020000088777201237, "Velocity"=4.8776402021072}, {"Time"=0.02400021077965827, "Velocity"=4.824438151461894}, {"Time"=0.028000421528213002, "Velocity"=4.762060561212428}, {"Time"=0.03200041540994551, "Velocity"=4.690758812947978}, {"Time"=0.036000063184231185, "Velocity"=4.610818448936833}, {"Time"=0.04000037297890258, "Velocity"=4.522533833672219}, {"Time"=0.044000423245738, "Velocity"=4.426272461056834}, {"Time"=0.04800029162553214, "Velocity"=4.322413668891642}, {"Time"=0.05200029270823189, "Velocity"=4.211359316208158}, {"Time"=0.05600001736121903, "Velocity"=4.093559370088427}, {"Time"=0.06000001293883861, "Velocity"=3.969462630827658}, {"Time"=0.0640004451707494, "Velocity"=3.839552128134903}, {"Time"=0.06800042472929116, "Velocity"=3.704369460181746}, {"Time"=0.07200014242532365, "Velocity"=3.564443048957042}, {"Time"=0.0760002580212144, "Velocity"=3.420301831449371}, {"Time"=0.0800000261763912, "Velocity"=3.272541369059561}, {"Time"=0.08400017452997474, "Velocity"=3.121717930556299}, {"Time"=0.08800015711169071, "Velocity"=2.968447067785735}, {"Time"=0.09200024710958415, "Velocity"=2.813323289411822}, {"Time"=0.09600046215012985, "Velocity"=2.6569580106916058}, {"Time"=0.10000038691637159, "Velocity"=2.499984622816152}, {"Time"=0.10400041106391561, "Velocity"=2.3430074006328305}, {"Time"=0.1080000261096995, "Velocity"=2.1866657027535057}, {"Time"=0.1120002228571225, "Velocity"=2.0315379156304476}, {"Time"=0.11600005865499748, "Velocity"=1.8782728454513444}, {"Time"=0.1200004797304372, "Velocity"=1.7274393882922903}, {"Time"=0.1240001629685658, "Velocity"=1.5796824569447379}, {"Time"=0.12800047848734047, "Velocity"=1.4355345573162932}, {"Time"=0.13200006589113764, "Velocity"=1.2956133355733332}, {"Time"=0.13600004001475047, "Velocity"=1.160431475645537}, {"Time"=0.14000034335462172, "Velocity"=1.0305257536216412}, {"Time"=0.14400035305963535, "Velocity"=0.9064291397205193}, {"Time"=0.14800042076334197, "Velocity"=0.7886199927738271}, {"Time"=0.15200029410138058, "Velocity"=0.6775703349762917}, {"Time"=0.15600031700604464, "Velocity"=0.5737087759380032}, {"Time"=0.16000029061770876, "Velocity"=0.47745063385170994}, {"Time"=0.16400020489267728, "Velocity"=0.389175714108094}, {"Time"=0.16800034082194923, "Velocity"=0.3092267039885715}, {"Time"=0.17200031966352872, "Velocity"=0.2379268899625615}, {"Time"=0.17600032146434255, "Velocity"=0.1755540195780829}, {"Time"=0.1800003096991534, "Velocity"=0.12235484927373219}, {"Time"=0.1840000857360056, "Velocity"=0.0785411761360237}, {"Time"=0.1880001992046059, "Velocity"=0.04428034288361315}, {"Time"=0.19200010865487005, "Velocity"=0.019712667897648063}, {"Time"=0.1960004663235367, "Velocity"=0.0049320066252910985}, {"Time"=0.20000041398843083, "Velocity"=5.5266913243923344e-11}, {"Time"=0.44142145663081306, "Velocity"=-3.562899519704275e-11}, {"Time"=0.4425929642321666, "Velocity"=-0.004933467625961054}, {"Time"=0.4437646237619058, "Velocity"=-0.019715279451253287}, {"Time"=0.4449361588925674, "Velocity"=-0.04428396435438883}, {"Time"=0.44610777338696483, "Velocity"=-0.07854626086349188}, {"Time"=0.44727922703474055, "Velocity"=-0.12235894380581175}, {"Time"=0.4484508917641267, "Velocity"=-0.17556359916009417}, {"Time"=0.4496224674612652, "Velocity"=-0.23793809870605087}, {"Time"=0.45079403762149745, "Velocity"=-0.30923960874635276}, {"Time"=0.4519656213693843, "Velocity"=-0.38918798554277406}, {"Time"=0.45313713408720246, "Velocity"=-0.4774613300717623}, {"Time"=0.45430877836574424, "Velocity"=-0.5737271351606212}, {"Time"=0.4554803018903897, "Velocity"=-0.6775849027795104}, {"Time"=0.4566519249073247, "Velocity"=-0.788644028823191}, {"Time"=0.4578234673935002, "Velocity"=-0.9064493537189756}, {"Time"=0.4589949643247566, "Velocity"=-1.030538427693559}, {"Time"=0.460166582811835, "Velocity"=-1.1604398043566868}, {"Time"=0.4613381653022563, "Velocity"=-1.2956239954752535}, {"Time"=0.46250980727229496, "Velocity"=-1.435568602403632}, {"Time"=0.4636813014253943, "Velocity"=-1.5796961022375458}, {"Time"=0.46485289063724405, "Velocity"=-1.7274672545946845}, {"Time"=0.46602449050426903, "Velocity"=-1.8782887095700955}, {"Time"=0.46719598746730157, "Velocity"=-2.0315503354979008}, {"Time"=0.4683676118484917, "Velocity"=-2.186677427786288}, {"Time"=0.4695391779377389, "Velocity"=-2.3430333697277113}, {"Time"=0.47071071058279595, "Velocity"=-2.5000042960331577}, {"Time"=0.47188235306988, "Velocity"=-2.6569899034859636}, {"Time"=0.47305388787911645, "Velocity"=-2.813341546741527}, {"Time"=0.47422550063648267, "Velocity"=-2.9684669201996563}, {"Time"=0.4753970287580537, "Velocity"=-3.121732351763251}, {"Time"=0.4765686401564869, "Velocity"=-3.2725548960332764}, {"Time"=0.4777402411961419, "Velocity"=-3.4203270272157353}, {"Time"=0.4789117541655816, "Velocity"=-3.564456189150118}, {"Time"=0.48008333092082317, "Velocity"=-3.704392352431738}, {"Time"=0.4812549728455815, "Velocity"=-3.8395826751457425}, {"Time"=0.4824264607400076, "Velocity"=-3.9694689463703066}, {"Time"=0.4835980064428127, "Velocity"=-4.093562707864842}, {"Time"=0.48476967393339215, "Velocity"=-4.211379599973376}, {"Time"=0.48594113809475903, "Velocity"=-4.322422706189478}, {"Time"=0.4871127188075141, "Velocity"=-4.426284837523065}, {"Time"=0.48828436744714, "Velocity"=-4.522550053883344}, {"Time"=0.48945588626203734, "Velocity"=-4.61082283017635}, {"Time"=0.4906275501240157, "Velocity"=-4.690775290140435}, {"Time"=0.49179911924232406, "Velocity"=-4.762075009618013}, {"Time"=0.49297067609945067, "Velocity"=-4.824446804295266}, {"Time"=0.4941422214339548, "Velocity"=-4.877644842478153}, {"Time"=0.4953138418232799, "Velocity"=-4.921462345979842}, {"Time"=0.4964854150390773, "Velocity"=-4.955721483588606}, {"Time"=0.4976569276834859, "Velocity"=-4.980287986695834}, {"Time"=0.49882846209618725, "Velocity"=-4.995067115337887}, {"Time"=0.5000000969848565, "Velocity"=-4.999999999966183}, {"Time"=0.5011715861981143, "Velocity"=-4.995066708766754}, {"Time"=0.5023432226274905, "Velocity"=-4.980285460844186}, {"Time"=0.5035147877129156, "Velocity"=-4.955716389833611}, {"Time"=0.5046864200688125, "Velocity"=-4.921453613635029}, {"Time"=0.5058578734380977, "Velocity"=-4.877640911790893}, {"Time"=0.5070295315847376, "Velocity"=-4.824436553719982}, {"Time"=0.5082011459378805, "Velocity"=-4.762059871343489}, {"Time"=0.5093726229966191, "Velocity"=-4.69076410806341}, {"Time"=0.5105442946986123, "Velocity"=-4.610809829650205}, {"Time"=0.5117157408409537, "Velocity"=-4.5225415199621875}, {"Time"=0.5128874192147183, "Velocity"=-4.426273041668763}, {"Time"=0.5140589497050069, "Velocity"=-4.322414647803724}, {"Time"=0.5152304559473024, "Velocity"=-4.211366905847879}, {"Time"=0.5164020719679304, "Velocity"=-4.093554607464228}, {"Time"=0.5175737335286933, "Velocity"=-3.9694478740775074}, {"Time"=0.5187452964304298, "Velocity"=-3.839552192031346}, {"Time"=0.5199168787402342, "Velocity"=-3.7043677189998436}, {"Time"=0.5210883531894858, "Velocity"=-3.564443165324585}, {"Time"=0.5222599350706716, "Velocity"=-3.4203050537104445}, {"Time"=0.5234315846129133, "Velocity"=-3.2725262348443867}, {"Time"=0.5246030544173771, "Velocity"=-3.1217215503036524}, {"Time"=0.525774720020729, "Velocity"=-2.9684378594215364}, {"Time"=0.5269462685833223, "Velocity"=-2.8133207343207167}, {"Time"=0.5281178284112066, "Velocity"=-2.6569656192691076}, {"Time"=0.5292893864502171, "Velocity"=-2.4999912862489744}, {"Time"=0.5304609731448376, "Velocity"=-2.3430131531739344}, {"Time"=0.5316324824384168, "Velocity"=-2.1866648858684896}, {"Time"=0.5328040896927567, "Velocity"=-2.031540173441984}, {"Time"=0.5339756699394806, "Velocity"=-1.8782678737580354}, {"Time"=0.535147319764835, "Velocity"=-1.7274404254572928}, {"Time"=0.5363187750324252, "Velocity"=-1.5796865709572114}, {"Time"=0.5374903342118713, "Velocity"=-1.4355514381573664}, {"Time"=0.5386619302803555, "Velocity"=-1.2956127653171532}, {"Time"=0.5398335411503904, "Velocity"=-1.160425771339298}, {"Time"=0.5410050851411254, "Velocity"=-1.030533062149048}, {"Time"=0.5421767252938255, "Velocity"=-0.9064294477320147}, {"Time"=0.5433482488434755, "Velocity"=-0.7886270468963448}, {"Time"=0.5445197747360768, "Velocity"=-0.6775778698945802}, {"Time"=0.5456914826059873, "Velocity"=-0.573704831705486}, {"Time"=0.5468629946245908, "Velocity"=-0.47745118658911534}, {"Time"=0.5480345468910789, "Velocity"=-0.3891758974445753}, {"Time"=0.5492061728253236, "Velocity"=-0.3092260156730008}, {"Time"=0.5503776383737377, "Velocity"=-0.23793205689992952}, {"Time"=0.551549250256696, "Velocity"=-0.1755565894679647}, {"Time"=0.5527208363301785, "Velocity"=-0.12235631849964569}, {"Time"=0.5538924418896343, "Velocity"=-0.07853908280343534}, {"Time"=0.5550639605644633, "Velocity"=-0.04428096317854631}, {"Time"=0.5562355962308128, "Velocity"=-0.019711582641101715}, {"Time"=0.5574071572620614, "Velocity"=-0.004932444826470117}, {"Time"=0.558578686689199, "Velocity"=-6.8882269681917525e-12}, {"Time"=0.9242645554782386, "Velocity"=-9.737506853680563e-12}, {"Time"=0.9299210829740109, "Velocity"=-0.004933047923986537}, {"Time"=0.9355780309236175, "Velocity"=-0.019713312479107094}, {"Time"=0.9412351082198321, "Velocity"=-0.04428313380367324}, {"Time"=0.9468919835079566, "Velocity"=-0.07854391784874565}, {"Time"=0.9525488339195877, "Velocity"=-0.12236094151588676}, {"Time"=0.958205469061791, "Velocity"=-0.17555920817180515}, {"Time"=0.9638622852492605, "Velocity"=-0.23793241189198133}, {"Time"=0.969519140223368, "Velocity"=-0.3092333627610564}, {"Time"=0.9751759539990372, "Velocity"=-0.389179658929095}, {"Time"=0.9808330670321187, "Velocity"=-0.47746116483175993}, {"Time"=0.9864895904937686, "Velocity"=-0.5737150030888363}, {"Time"=0.9921464288763495, "Velocity"=-0.6775761064849879}, {"Time"=0.9978038110945824, "Velocity"=-0.7886404532611914}, {"Time"=1.0034606176731187, "Velocity"=-0.9064476992448258}, {"Time"=1.0091173515884027, "Velocity"=-1.0305422305454124}, {"Time"=1.0147740433571775, "Velocity"=-1.1604348062310965}, {"Time"=1.0204308799169033, "Velocity"=-1.2956172540212705}, {"Time"=1.0260874598398804, "Velocity"=-1.435546373061055}, {"Time"=1.0317445126058686, "Velocity"=-1.5796882053319927}, {"Time"=1.0374017304979446, "Velocity"=-1.7274667038861666}, {"Time"=1.0430585435333806, "Velocity"=-1.8782835417531407}, {"Time"=1.0487150409372261, "Velocity"=-2.031545365770292}, {"Time"=1.054372136218472, "Velocity"=-2.1866722042234956}, {"Time"=1.0600288839005212, "Velocity"=-2.343026076733983}, {"Time"=1.0656859041676396, "Velocity"=-2.500006999492344}, {"Time"=1.0713428971621144, "Velocity"=-2.6569871388125534}, {"Time"=1.0769996833561033, "Velocity"=-2.813341994005756}, {"Time"=1.0826564402538648, "Velocity"=-2.968459462011321}, {"Time"=1.0883131677732139, "Velocity"=-3.1217274077826884}, {"Time"=1.0939698498803552, "Velocity"=-3.272540589839043}, {"Time"=1.0996267663131298, "Velocity"=-3.42031114209771}, {"Time"=1.1052836631976901, "Velocity"=-3.5644490753217983}, {"Time"=1.1109406455163595, "Velocity"=-3.7043881294407965}, {"Time"=1.1165973827015423, "Velocity"=-3.839568050908669}, {"Time"=1.1222540088584654, "Velocity"=-3.9694590331496347}, {"Time"=1.1279108599734708, "Velocity"=-4.093556011875631}, {"Time"=1.1335680721774604, "Velocity"=-4.211371268444823}, {"Time"=1.1392246366560763, "Velocity"=-4.3224193568984175}, {"Time"=1.1448816691505646, "Velocity"=-4.426284208369835}, {"Time"=1.1505386660030763, "Velocity"=-4.522545834545664}, {"Time"=1.1561955001824018, "Velocity"=-4.610822572696121}, {"Time"=1.1618523282590345, "Velocity"=-4.690768834968408}, {"Time"=1.1675094555121592, "Velocity"=-4.762072749630675}, {"Time"=1.1731660976942915, "Velocity"=-4.824443475747124}, {"Time"=1.1788226642575772, "Velocity"=-4.877640723015898}, {"Time"=1.1844798914521508, "Velocity"=-4.9214600236396}, {"Time"=1.19013649791727, "Velocity"=-4.955718437273642}, {"Time"=1.1957934778179877, "Velocity"=-4.980287399391089}, {"Time"=1.2014499296310812, "Velocity"=-4.995066443663182}, {"Time"=1.207107431167707, "Velocity"=-4.9999999999713305}, {"Time"=1.212763784235413, "Velocity"=-4.9950669425629854}, {"Time"=1.2184205374727226, "Velocity"=-4.98028734617634}, {"Time"=1.22407785383885, "Velocity"=-4.9557166070009675}, {"Time"=1.2297342292622846, "Velocity"=-4.9214591900397835}, {"Time"=1.2353913731832697, "Velocity"=-4.877640401742916}, {"Time"=1.2410483527254181, "Velocity"=-4.824438871515822}, {"Time"=1.2467054177658237, "Velocity"=-4.762062424822361}, {"Time"=1.2523621444982755, "Velocity"=-4.690762510720646}, {"Time"=1.2580189080791506, "Velocity"=-4.610816498232076}, {"Time"=1.2636757091731374, "Velocity"=-4.522539711058972}, {"Time"=1.2693327883461103, "Velocity"=-4.426276110659624}, {"Time"=1.2749893180324714, "Velocity"=-4.322420218202914}, {"Time"=1.2806464511512656, "Velocity"=-4.211360675206888}, {"Time"=1.2863028767774773, "Velocity"=-4.0935616442569565}, {"Time"=1.2919598376147243, "Velocity"=-3.9694624821016715}, {"Time"=1.2976170509327392, "Velocity"=-3.839557884204176}, {"Time"=1.303273368718014, "Velocity"=-3.7043877830718186}, {"Time"=1.308930216784107, "Velocity"=-3.5644520908083517}, {"Time"=1.3145876487652737, "Velocity"=-3.420300425571659}, {"Time"=1.3202441942357528, "Velocity"=-3.272539424778275}, {"Time"=1.3259010454799944, "Velocity"=-3.121721672201785}, {"Time"=1.3315579126406758, "Velocity"=-2.9684498364001417}, {"Time"=1.3372149253825931, "Velocity"=-2.813325223826799}, {"Time"=1.3428712982102293, "Velocity"=-2.656981724415714}, {"Time"=1.3485287004451476, "Velocity"=-2.499990210592372}, {"Time"=1.3541851827943705, "Velocity"=-2.343024228403295}, {"Time"=1.359842523760424, "Velocity"=-2.186654022428241}, {"Time"=1.3654987996160721, "Velocity"=-2.031549714866233}, {"Time"=1.3711561521224245, "Velocity"=-1.8782648316495862}, {"Time"=1.3768130680967168, "Velocity"=-1.727445613838503}, {"Time"=1.3824697235007897, "Velocity"=-1.5796821095215876}, {"Time"=1.3881261856360543, "Velocity"=-1.4355552805670915}, {"Time"=1.393783389778028, "Velocity"=-1.2956106914562442}, {"Time"=1.3994402117070435, "Velocity"=-1.1604288261723106}, {"Time"=1.4050973266685909, "Velocity"=-1.0305269936500012}, {"Time"=1.4107537615737404, "Velocity"=-0.9064395850078305}, {"Time"=1.4164109244364238, "Velocity"=-0.7886255646252787}, {"Time"=1.4220677729292772, "Velocity"=-0.6775722704692798}, {"Time"=1.4277241582867912, "Velocity"=-0.573719449674576}, {"Time"=1.4333811094829563, "Velocity"=-0.4774582838115842}, {"Time"=1.439038015998405, "Velocity"=-0.3891801053324633}, {"Time"=1.444694734035628, "Velocity"=-0.30923504484422437}, {"Time"=1.450351914306421, "Velocity"=-0.23793005254095556}, {"Time"=1.4560088613288062, "Velocity"=-0.17555583090113397}, {"Time"=1.461665488975964, "Velocity"=-0.12235817080759148}, {"Time"=1.4673227116110588, "Velocity"=-0.07853911763439032}, {"Time"=1.472979285616935, "Velocity"=-0.044281084583606904}, {"Time"=1.4786361671612562, "Velocity"=-0.019712623097946563}, {"Time"=1.4842930505551715, "Velocity"=-0.004932815112555703}, {"Time"=1.4899499591723449, "Velocity"=-1.0696527286538092e-11}]}]
  out "XY Graph":cluster{"X":dbl, "Y":dbl}[](graph)=[{"X"=0.0, "Y"=0.0}, {"X"=0.0, "Y"=0.5}, {"X"=0.5, "Y"=1.0}, {"X"=1.0, "Y"=0.5}, {"X"=0.5, "Y"=0.0}, {"X"=0.0, "Y"=0.5}]
  in  "Acceleration Max":dbl=5.0
  in  "Velocity":dbl=1.0
  in  "LineArray":cluster{"X":dbl, "Y":dbl, "OnOff":bool}[](array[cluster])=[{"X"=0.0, "Y"=0.0, "OnOff"=FALSE}, {"X"=0.0, "Y"=0.5, "OnOff"=FALSE}, {"X"=0.5, "Y"=1.0, "OnOff"=FALSE}, {"X"=1.0, "Y"=0.5, "OnOff"=FALSE}, {"X"=0.5, "Y"=0.0, "OnOff"=FALSE}, {"X"=0.0, "Y"=0.5, "OnOff"=FALSE}, {"X"=0.0, "Y"=0.0, "OnOff"=FALSE}]
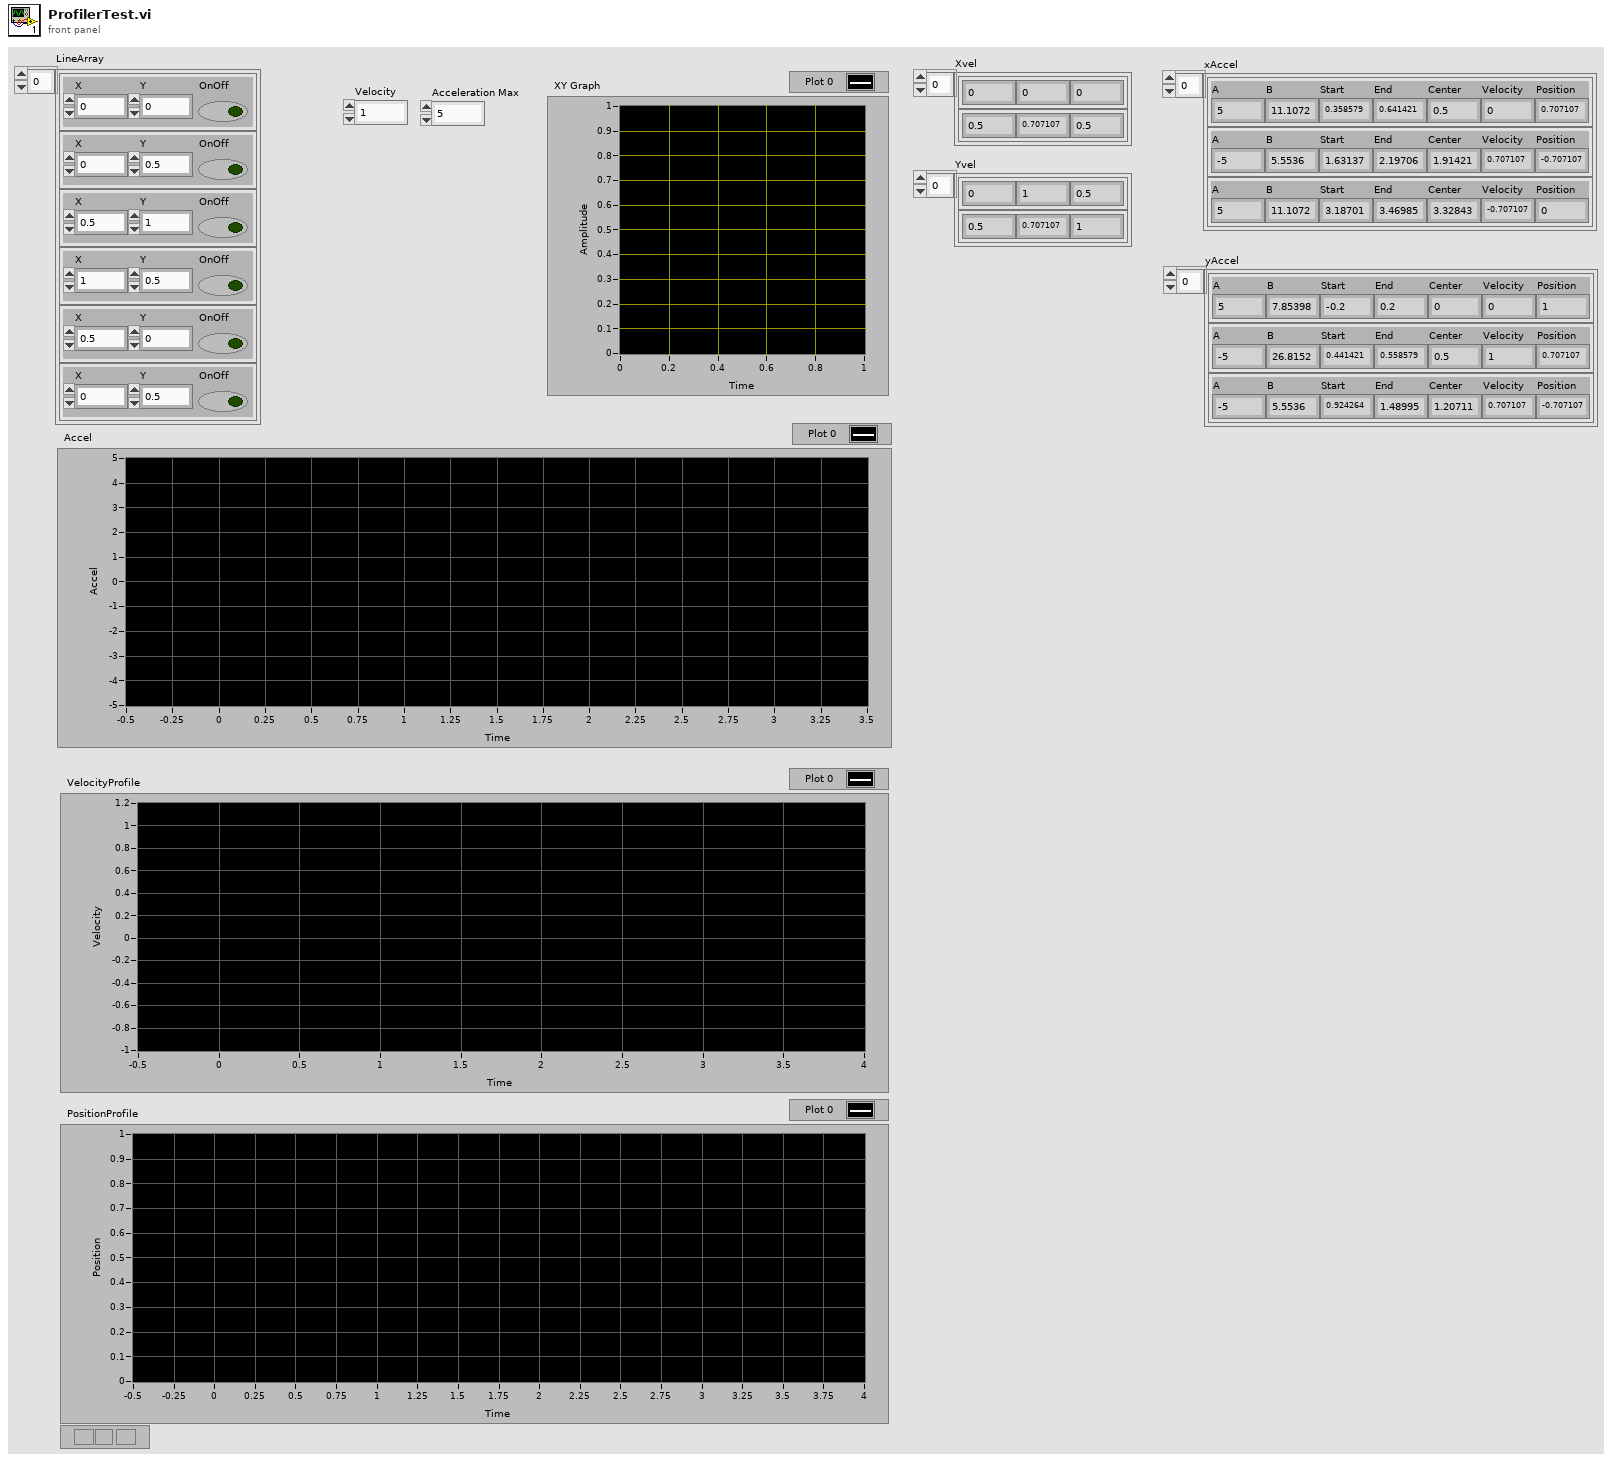
[diagram p1: front panel]
types:
  T1 = cluster{cluster{"Time":dbl, "delVelocity":dbl}[]}[]
  T2 = cluster{"A":dbl, "B":dbl, "Start":dbl, "End":dbl, "Center":dbl, "Velocity":dbl, "Position":dbl}[]
  T3 = cluster{cluster{"Time":dbl, "delVelocity":dbl}[]}
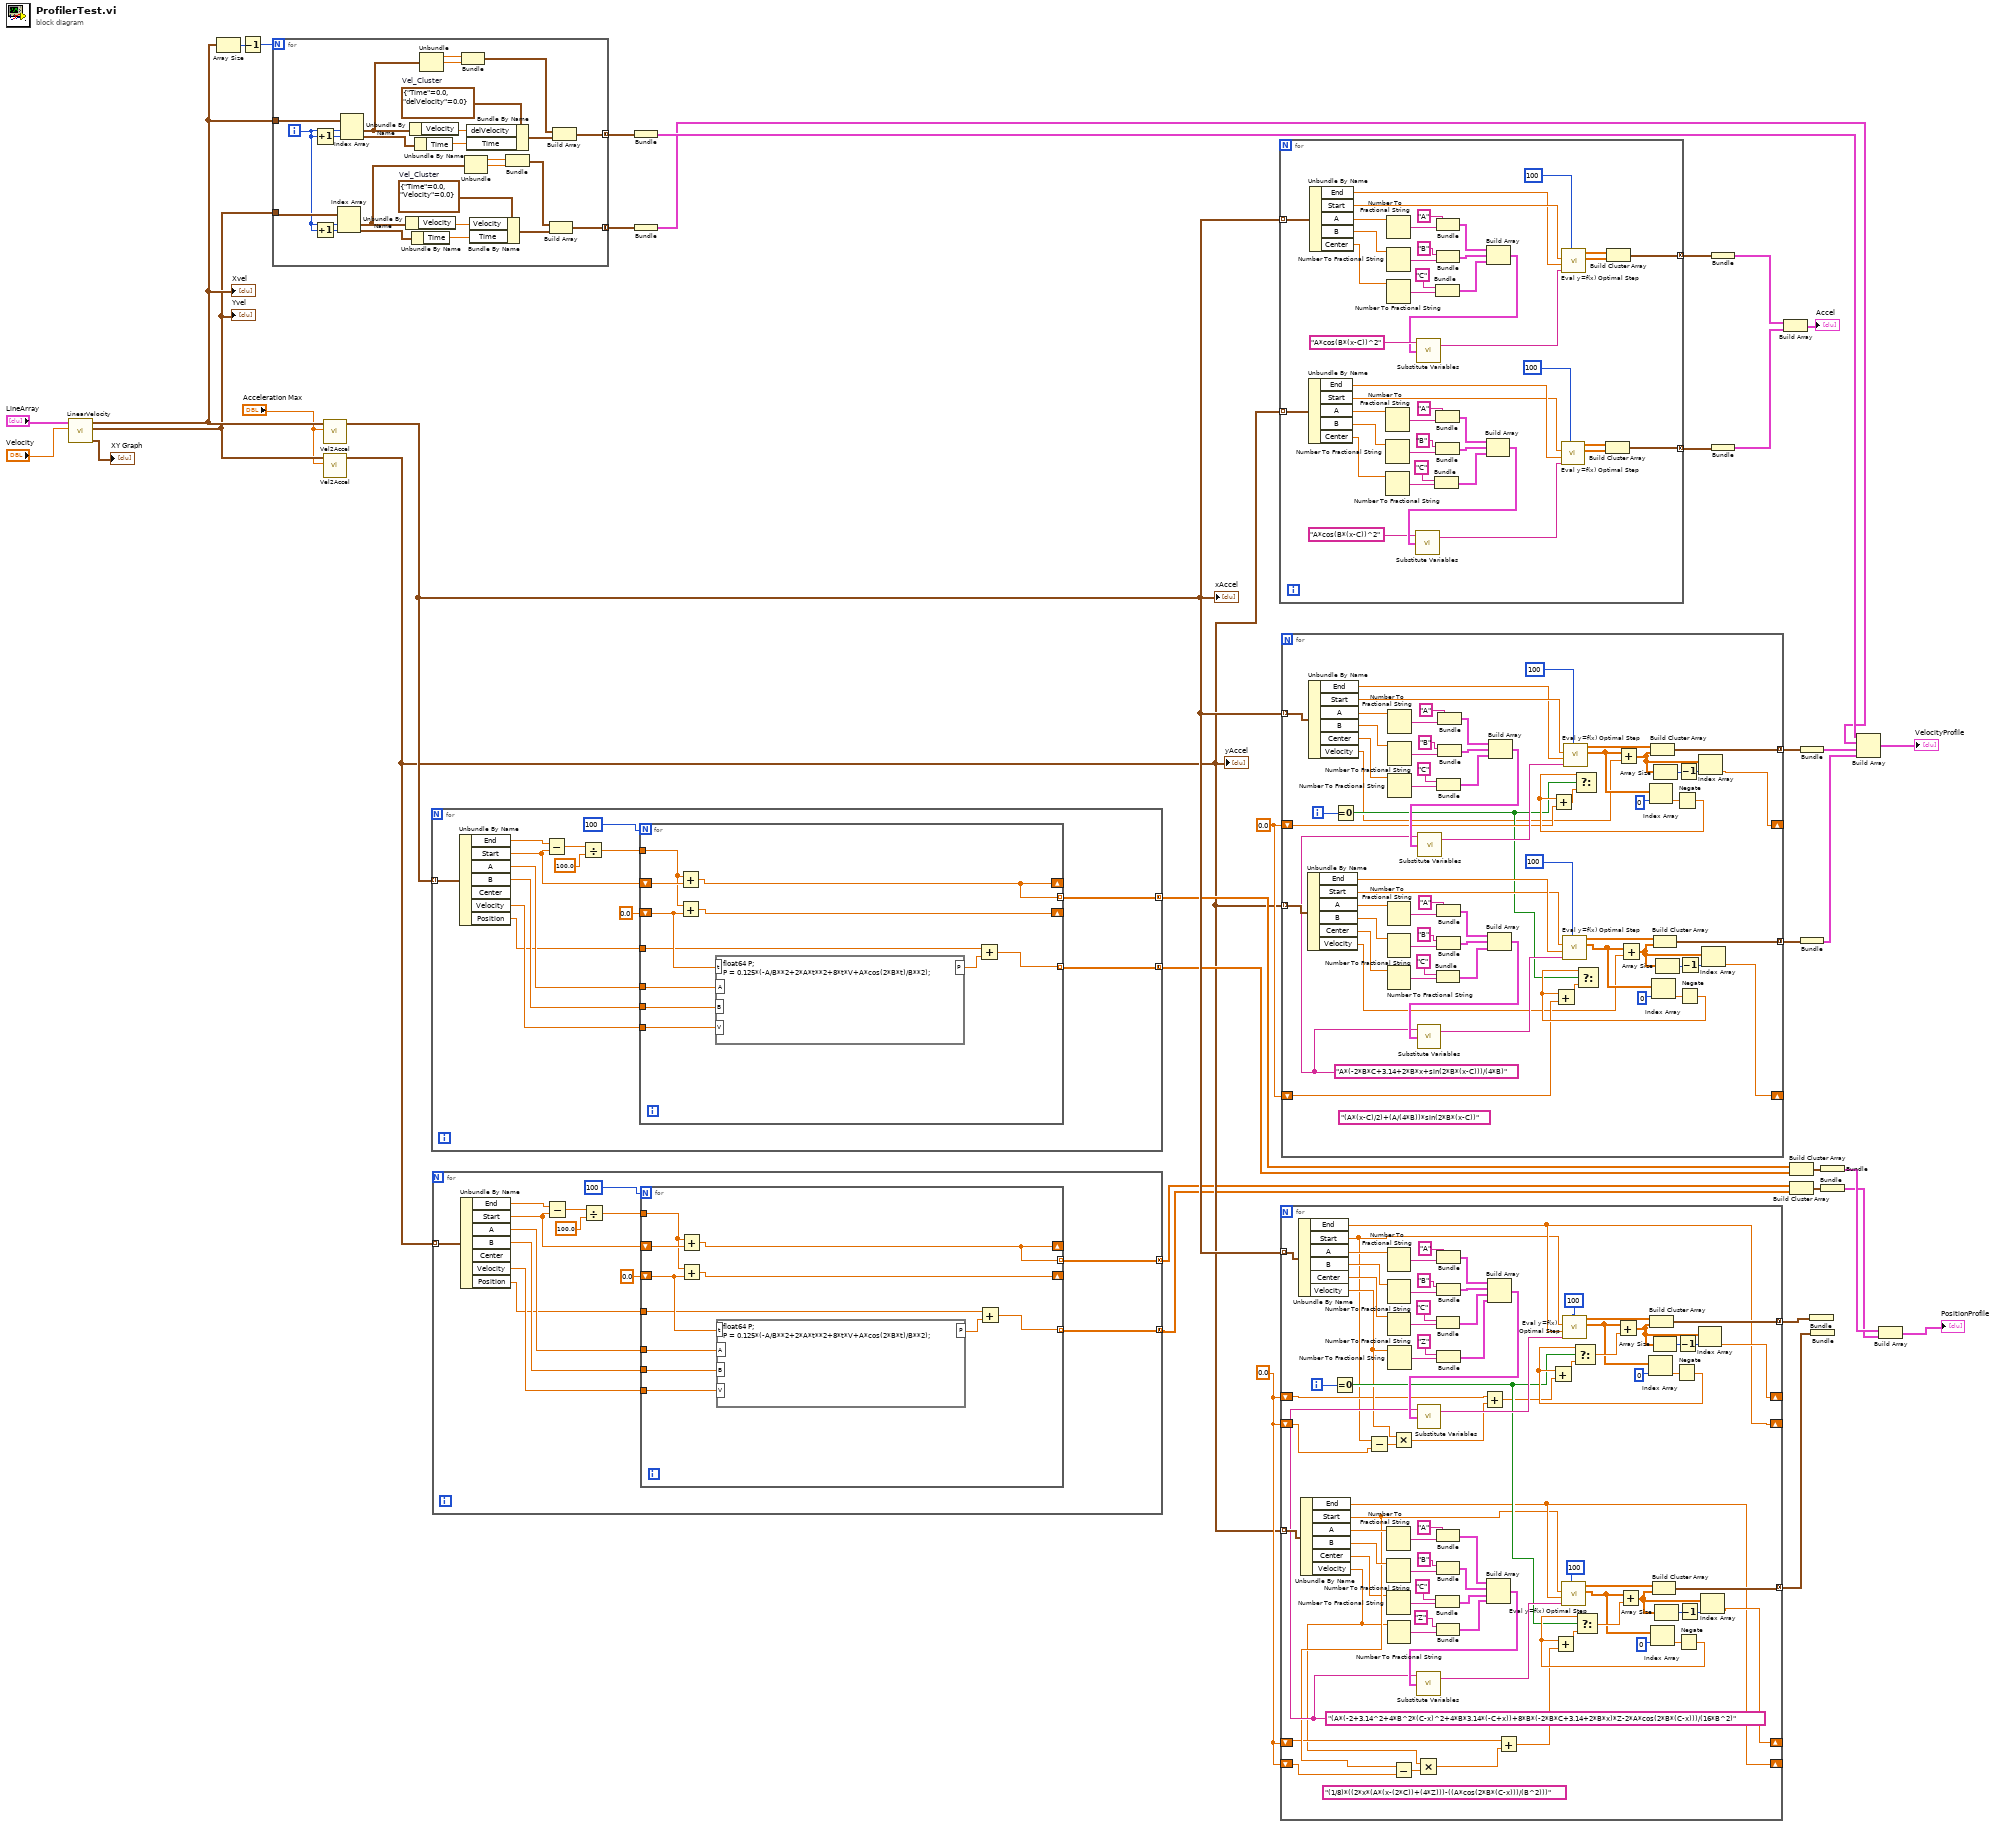
[diagram p0: block diagram]
diagram:
  w18 = 0.0
  w28 = 0.0
  n1 = call "LinearVelocity.vi"("Velocity"="Velocity", "LineArray"="LineArray") -> ("XY Graph"=→"XY Graph":cluster{"X":dbl, "Y":dbl}[], "Yvelocities"=w12:cluster{"Time":dbl, "Velocity":dbl, "Y":dbl}[], "Xvelocities"=w13:cluster{"Time":dbl, "Velocity":dbl, "X":dbl}[])  [unwired: 7 in]
  "Xvel" <- w13
  "Yvel" <- w12
  n2 = Array Size(array=w13) -> (size(s)=w37:i32)
  n3 = Decrement(x=w37) -> (x-1=w36:i32)
  n4 = for {
    N: w36 -> [_]
    tunnel: w13 -> [w57]
    tunnel: w12 -> [w48]
    tunnel: [w55] -> w35 mode=concatenating
    tunnel: [w46] -> w34 mode=concatenating
    i -> [w47]
    w51 = cluster{"Time":dbl, "Velocity":dbl} {"Time"=0.0, "Velocity"=0.0}  # Vel_Cluster
    w60 = cluster{"Time":dbl, "delVelocity":dbl} {"Time"=0.0, "delVelocity"=0.0}  # Vel_Cluster
    n5 = Increment(x=w47) -> (x+1=w62:i32)
    n6 = Increment(x=w47) -> (x+1=w49:i32)
    n7 = Index Array(array=w48, index #1=w47, index #2=w49) -> (element #1=w38:cluster{"Time":dbl, "Velocity":dbl, "Y":dbl}, element #2=w50:cluster{"Time":dbl, "Velocity":dbl, "Y":dbl})
    n8 = Index Array(array=w57, index #1=w47, index #2=w62) -> (element #1=w45:cluster{"Time":dbl, "Velocity":dbl, "X":dbl}, element #2=w61:cluster{"Time":dbl, "Velocity":dbl, "X":dbl})
    n9 = Unbundle By Name(w38) -> ("Velocity"=w52:dbl)
    n10 = Unbundle By Name(w45) -> ("Velocity"=w59:dbl)
    n11 = Unbundle By Name(w50) -> ("Time"=w53:dbl)
    n12 = Unbundle By Name(w61) -> ("Time"=w58:dbl)
    n13 = Unbundle(w45) -> ("Time"=w44:dbl, "Velocity"=w43:dbl)  [unwired: 1 out]
    n14 = Bundle("Time"=w44, "Velocity"=w43) -> (w42:cluster{"Time":dbl, "Velocity":dbl})  [unwired: 1 in]
    n15 = Unbundle(w38) -> ("Time"=w40:dbl, "Velocity"=w41:dbl)  [unwired: 1 out]
    n16 = Bundle By Name(cluster=w60, "delVelocity"=w59, "Time"=w58) -> (w56:cluster{"Time":dbl, "delVelocity":dbl})
    n17 = Bundle By Name(cluster=w51, "Velocity"=w52, "Time"=w53) -> (w54:cluster{"Time":dbl, "Velocity":dbl})
    n18 = Bundle("Time"=w40, "Velocity"=w41) -> (w39:cluster{"Time":dbl, "Velocity":dbl})  [unwired: 1 in]
    n19 = Build Array(w39, w54) -> (w46:cluster{"Time":dbl, "Velocity":dbl}[])
    n20 = Build Array(w42, w56) -> (w55:cluster{"Time":dbl, "delVelocity":dbl}[])
  }
  n21 = call "Vel2Accel.vi"("Acceleration Max"="Acceleration Max", "Velocities"=w13) -> ("AccelParams"=w10:T2)  [unwired: 9 in]
  "xAccel" <- w10
  n22 = call "Vel2Accel.vi"("Acceleration Max"="Acceleration Max", "Velocities"=w12) -> ("AccelParams"=w5:T2)  [unwired: 9 in]
  "yAccel" <- w5
  n23 = for {
    tunnel: w10 -> [w76] mode=indexing
    tunnel: [w69] -> w9 mode=concatenating
    tunnel: [w68] -> w8 mode=concatenating
    n24 = Unbundle By Name(w76) -> ("End"=w66:dbl, "Start"=w65:dbl, "A"=w72:dbl, "B"=w71:dbl, "Velocity"=w70:dbl, "Position"=w64:dbl)  [unwired: 1 out]
    n25 = Subtract(x=w66, y=w65) -> (x-y=w75:dbl)
    n26 = Divide(x=w75, y=100.0) -> (x/y=w73:dbl)
    n27 = for {
      N: 100 -> [_]
      shift-right: [w78] -> _
      shift-left: w65 -> [w87]
      tunnel: w73 -> [w86]
      shift-right: [w85] -> _
      shift-left: 0.0 -> [w84]
      tunnel: w72 -> [w83]
      tunnel: w71 -> [w82]
      tunnel: w70 -> [w81]
      tunnel: w64 -> [w79]
      tunnel: [w77] -> w68 mode=indexing
      tunnel: [w78] -> w69 mode=indexing
      n28 = Add(x=w86, y=w87) -> (x+y=w78:dbl)
      n29 = Add(x=w86, y=w84) -> (x+y=w85:dbl)
      n30 = formula code="float64 P;\nP = 0.125*(-A/B**2+2*A*t**2+8*t*V+A*cos(2*B*t)/B**2);"("A"=w83, "B"=w82, "V"=w81, "t"=w84) -> ("P"=w80:dbl)
      n31 = Add(x=w79, y=w80) -> (x+y=w77:dbl)
    }
  }
  n32 = for {
    tunnel: w5 -> [w101] mode=indexing
    tunnel: [w94] -> w3 mode=concatenating
    tunnel: [w93] -> w2 mode=concatenating
    n33 = Unbundle By Name(w101) -> ("End"=w91:dbl, "Start"=w90:dbl, "A"=w97:dbl, "B"=w96:dbl, "Velocity"=w95:dbl, "Position"=w89:dbl)  [unwired: 1 out]
    n34 = Subtract(x=w91, y=w90) -> (x-y=w100:dbl)
    n35 = Divide(x=w100, y=100.0) -> (x/y=w98:dbl)
    n36 = for {
      N: 100 -> [_]
      shift-right: [w103] -> _
      shift-left: w90 -> [w112]
      tunnel: w98 -> [w111]
      shift-right: [w110] -> _
      shift-left: 0.0 -> [w109]
      tunnel: w97 -> [w108]
      tunnel: w96 -> [w107]
      tunnel: w95 -> [w106]
      tunnel: w89 -> [w104]
      tunnel: [w102] -> w93 mode=indexing
      tunnel: [w103] -> w94 mode=indexing
      n37 = Add(x=w111, y=w112) -> (x+y=w103:dbl)
      n38 = Add(x=w111, y=w109) -> (x+y=w110:dbl)
      n39 = formula code="float64 P;\nP = 0.125*(-A/B**2+2*A*t**2+8*t*V+A*cos(2*B*t)/B**2);"("A"=w108, "B"=w107, "V"=w106, "t"=w109) -> ("P"=w105:dbl)
      n40 = Add(x=w104, y=w105) -> (x+y=w102:dbl)
    }
  }
  n41 = Bundle(w35) -> (w23:T3)  [unwired: 1 in]
  n42 = Bundle(w34) -> (w22:cluster{cluster{"Time":dbl, "Velocity":dbl}[]})  [unwired: 1 in]
  n43 = for {
    tunnel: w10 -> [w156] mode=indexing
    tunnel: [w135] -> w32 mode=concatenating
    tunnel: w5 -> [w114] mode=indexing
    tunnel: [w113] -> w30 mode=concatenating
    n44 = Unbundle By Name(w114) -> ("End"=w131:dbl, "Start"=w130:dbl, "A"=w116:dbl, "B"=w117:dbl, "Center"=w118:dbl)
    n45 = Unbundle By Name(w156) -> ("End"=w139:dbl, "Start"=w140:dbl, "A"=w154:dbl, "B"=w153:dbl, "Center"=w152:dbl)
    n46 = Number To Fractional String(number=w116) -> (F-format string=w119:string)  [unwired: 3 in]
    n47 = Number To Fractional String(number=w117) -> (F-format string=w121:string)  [unwired: 3 in]
    n48 = Number To Fractional String(number=w118) -> (F-format string=w124:string)  [unwired: 3 in]
    n49 = Number To Fractional String(number=w154) -> (F-format string=w151:string)  [unwired: 3 in]
    n50 = Number To Fractional String(number=w153) -> (F-format string=w149:string)  [unwired: 3 in]
    n51 = Number To Fractional String(number=w152) -> (F-format string=w146:string)  [unwired: 3 in]
    n52 = Bundle("C", w124) -> (w127:cluster{string, string})  [unwired: 1 in]
    n53 = Bundle("C", w146) -> (w143:cluster{string, string})  [unwired: 1 in]
    n54 = Bundle("A", w119) -> (w125:cluster{string, string})  [unwired: 1 in]
    n55 = Bundle("B", w121) -> (w126:cluster{string, string})  [unwired: 1 in]
    n56 = Bundle("A", w151) -> (w145:cluster{string, string})  [unwired: 1 in]
    n57 = Bundle("B", w149) -> (w144:cluster{string, string})  [unwired: 1 in]
    n58 = Build Array(w125, w126, w127) -> (w128:cluster{string, string}[])
    n59 = call <vilib>:"Substitute Variables.vi"("Substitution Rules"=w128, "original formula"="A*cos(B*(x-C))^2") -> ("formula after substitution"=w129:string)  [unwired: 1 in, 1 out]
    n60 = Build Array(w145, w144, w143) -> (w142:cluster{string, string}[])
    n61 = call <vilib>:"Substitute Variables.vi"("Substitution Rules"=w142, "original formula"="A*cos(B*(x-C))^2") -> ("formula after substitution"=w141:string)  [unwired: 1 in, 1 out]
    n62 = call <vilib>:"Eval y=f(x) Optimal Step.vi"("number of points"=u32 100, "formula"=w129, "end"=w131, "start"=w130) -> ("Y Values"=w134:dbl[], "X Values"=w133:dbl[])  [unwired: 1 in, 2 out]
    n63 = call <vilib>:"Eval y=f(x) Optimal Step.vi"("number of points"=u32 100, "formula"=w141, "end"=w139, "start"=w140) -> ("Y Values"=w136:dbl[], "X Values"=w137:dbl[])  [unwired: 1 in, 2 out]
    n64 = Build Cluster Array(w133, w134) -> (w113:cluster{dbl, dbl}[])
    n65 = Build Cluster Array(w137, w136) -> (w135:cluster{dbl, dbl}[])
  }
  n66 = for {
    tunnel: w10 -> [w237] mode=indexing
    tunnel: [w220] -> w20 mode=concatenating
    tunnel: w5 -> [w205] mode=indexing
    tunnel: [w188] -> w19 mode=concatenating
    shift-right: [w175] -> _
    shift-left: w18 -> [w169]
    shift-right: [w166] -> _
    shift-left: w18 -> [w161]
    shift-right: [w174] -> _
    shift-left: w18 -> [w168]
    shift-right: [w165] -> _
    shift-left: w18 -> [w163]
    i -> [w202]
    (unwired) "(1/8)*((2*x*(A*(x-(2*C))+(4*Z)))-((A*cos(2*B*(C-x)))/(B^2)))"
    w204 = "(A*(-2+3.14^2+4*B^2*(C-x)^2+4*B*3.14*(-C+x))+8*B*(-2*B*C+3.14+2*B*x)*Z-2*A*cos(2*B*(C-x)))/(16*B^2)"
    n67 = Unbundle By Name(w237) -> ("End"=w174:dbl, "Start"=w167:dbl, "A"=w236:dbl, "B"=w235:dbl, "Center"=w234:dbl, "Velocity"=w172:dbl)
    n68 = Unbundle By Name(w205) -> ("End"=w165:dbl, "Start"=w162:dbl, "A"=w206:dbl, "B"=w207:dbl, "Center"=w157:dbl, "Velocity"=w158:dbl)
    n69 = Equal To 0?(x=w202) -> (x = 0?=w189:bool)
    n70 = Subtract(x=w167, y=w168) -> (x-y=w173:dbl)
    n71 = Number To Fractional String(number=w206) -> (F-format string=w208:string)  [unwired: 3 in]
    n72 = Number To Fractional String(number=w207) -> (F-format string=w210:string)  [unwired: 3 in]
    n73 = Number To Fractional String(number=w157) -> (F-format string=w213:string)  [unwired: 3 in]
    n74 = Number To Fractional String(number=w236) -> (F-format string=w233:string)  [unwired: 3 in]
    n75 = Number To Fractional String(number=w235) -> (F-format string=w231:string)  [unwired: 3 in]
    n76 = Number To Fractional String(number=w234) -> (F-format string=w228:string)  [unwired: 3 in]
    n77 = Number To Fractional String(number=w158) -> (F-format string=w182:string)  [unwired: 3 in]
    n78 = Number To Fractional String(number=w172) -> (F-format string=w185:string)  [unwired: 3 in]
    n79 = Multiply(x=w172, y=w173) -> (x*y=w170:dbl)
    n80 = Subtract(x=w162, y=w163) -> (x-y=w164:dbl)
    n81 = Multiply(x=w158, y=w164) -> (x*y=w159:dbl)
    n82 = Bundle("C", w213) -> (w216:cluster{string, string})  [unwired: 1 in]
    n83 = Bundle("C", w228) -> (w225:cluster{string, string})  [unwired: 1 in]
    n84 = Bundle("A", w208) -> (w214:cluster{string, string})  [unwired: 1 in]
    n85 = Bundle("B", w210) -> (w215:cluster{string, string})  [unwired: 1 in]
    n86 = Bundle("Z", w182) -> (w180:cluster{string, string})  [unwired: 1 in]
    n87 = Bundle("A", w233) -> (w227:cluster{string, string})  [unwired: 1 in]
    n88 = Bundle("B", w231) -> (w226:cluster{string, string})  [unwired: 1 in]
    n89 = Bundle("Z", w185) -> (w183:cluster{string, string})  [unwired: 1 in]
    n90 = Add(x=w169, y=w170) -> (x+y=w171:dbl)
    n91 = Build Array(w214, w215, w216, w180) -> (w217:cluster{string, string}[])
    n92 = call <vilib>:"Substitute Variables.vi"("Substitution Rules"=w217, "original formula"=w204) -> ("formula after substitution"=w218:string)  [unwired: 1 in, 1 out]
    n93 = Build Array(w227, w226, w225, w183) -> (w224:cluster{string, string}[])
    n94 = call <vilib>:"Substitute Variables.vi"("Substitution Rules"=w224, "original formula"=w204) -> ("formula after substitution"=w223:string)  [unwired: 1 in, 1 out]
    n95 = Add(x=w161, y=w159) -> (x+y=w160:dbl)
    n96 = call <vilib>:"Eval y=f(x) Optimal Step.vi"("number of points"=u32 100, "formula"=w218, "end"=w165, "start"=w162) -> ("Y Values"=w178:dbl[], "X Values"=w190:dbl[])  [unwired: 1 in, 2 out]
    n97 = call <vilib>:"Eval y=f(x) Optimal Step.vi"("number of points"=u32 100, "formula"=w223, "end"=w174, "start"=w167) -> ("Y Values"=w179:dbl[], "X Values"=w221:dbl[])  [unwired: 1 in, 2 out]
    n98 = Index Array(array=w179, index=0) -> (element=w197:dbl)
    n99 = Index Array(array=w178, index=0) -> (element=w195:dbl)
    n100 = Negate(x=w197) -> (-x=w201:dbl)
    n101 = Add(x=w201, y=w171) -> (x+y=w200:dbl)
    n102 = Select(t=w201, s=w189, f=w200) -> (s? t:f=w203:dbl)
    n103 = Add(x=w179, y=w203) -> (x+y=w177:dbl[])
    n104 = Build Cluster Array(w221, w177) -> (w220:cluster{dbl, dbl}[])
    n105 = Array Size(array=w177) -> (size(s)=w199:i32)
    n106 = Decrement(x=w199) -> (x-1=w196:i32)
    n107 = Negate(x=w195) -> (-x=w192:dbl)
    n108 = Add(x=w192, y=w160) -> (x+y=w193:dbl)
    n109 = Select(t=w192, s=w189, f=w193) -> (s? t:f=w191:dbl)
    n110 = Add(x=w178, y=w191) -> (x+y=w176:dbl[])
    n111 = Build Cluster Array(w190, w176) -> (w188:cluster{dbl, dbl}[])
    n112 = Array Size(array=w176) -> (size(s)=w186:i32)
    n113 = Decrement(x=w186) -> (x-1=w187:i32)
    n114 = Index Array(array=w177, index=w196) -> (element=w175:dbl)
    n115 = Index Array(array=w176, index=w187) -> (element=w166:dbl)
  }
  n116 = for {
    tunnel: w10 -> [w302] mode=indexing
    tunnel: [w283] -> w27 mode=concatenating
    tunnel: w5 -> [w265] mode=indexing
    tunnel: [w246] -> w17 mode=concatenating
    shift-right: [w255] -> _
    shift-left: w28 -> [w260]
    shift-right: [w242] -> _
    shift-left: w28 -> [w241]
    i -> [w263]
    w240 = "A*(-2*B*C+3.14+2*B*x+sin(2*B*(x-C)))/(4*B)"
    (unwired) "(A*(x-C)/2)+(A/(4*B))*sin(2*B*(x-C))"
    n117 = Unbundle By Name(w265) -> ("End"=w281:dbl, "Start"=w280:dbl, "A"=w266:dbl, "B"=w267:dbl, "Center"=w268:dbl, "Velocity"=w238:dbl)
    n118 = Unbundle By Name(w302) -> ("End"=w286:dbl, "Start"=w287:dbl, "A"=w301:dbl, "B"=w300:dbl, "Center"=w299:dbl, "Velocity"=w239:dbl)
    n119 = Equal To 0?(x=w263) -> (x = 0?=w247:bool)
    n120 = Number To Fractional String(number=w266) -> (F-format string=w269:string)  [unwired: 3 in]
    n121 = Number To Fractional String(number=w267) -> (F-format string=w271:string)  [unwired: 3 in]
    n122 = Number To Fractional String(number=w268) -> (F-format string=w274:string)  [unwired: 3 in]
    n123 = Number To Fractional String(number=w301) -> (F-format string=w298:string)  [unwired: 3 in]
    n124 = Number To Fractional String(number=w300) -> (F-format string=w296:string)  [unwired: 3 in]
    n125 = Number To Fractional String(number=w299) -> (F-format string=w293:string)  [unwired: 3 in]
    n126 = Bundle("C", w274) -> (w277:cluster{string, string})  [unwired: 1 in]
    n127 = Bundle("C", w293) -> (w290:cluster{string, string})  [unwired: 1 in]
    n128 = Bundle("A", w269) -> (w275:cluster{string, string})  [unwired: 1 in]
    n129 = Bundle("B", w271) -> (w276:cluster{string, string})  [unwired: 1 in]
    n130 = Bundle("A", w298) -> (w292:cluster{string, string})  [unwired: 1 in]
    n131 = Bundle("B", w296) -> (w291:cluster{string, string})  [unwired: 1 in]
    n132 = Build Array(w275, w276, w277) -> (w278:cluster{string, string}[])
    n133 = call <vilib>:"Substitute Variables.vi"("Substitution Rules"=w278, "original formula"=w240) -> ("formula after substitution"=w279:string)  [unwired: 1 in, 1 out]
    n134 = Build Array(w292, w291, w290) -> (w289:cluster{string, string}[])
    n135 = call <vilib>:"Substitute Variables.vi"("Substitution Rules"=w289, "original formula"=w240) -> ("formula after substitution"=w288:string)  [unwired: 1 in, 1 out]
    n136 = call <vilib>:"Eval y=f(x) Optimal Step.vi"("number of points"=u32 100, "formula"=w279, "end"=w281, "start"=w280) -> ("Y Values"=w248:dbl[], "X Values"=w249:dbl[])  [unwired: 1 in, 2 out]
    n137 = call <vilib>:"Eval y=f(x) Optimal Step.vi"("number of points"=u32 100, "formula"=w288, "end"=w286, "start"=w287) -> ("Y Values"=w264:dbl[], "X Values"=w284:dbl[])  [unwired: 1 in, 2 out]
    n138 = Add(x=w264, y=w239) -> (x+y=w254:dbl[])
    n139 = Add(x=w248, y=w238) -> (x+y=w245:dbl[])
    n140 = Index Array(array=w264, index=0) -> (element=w257:dbl)
    n141 = Build Cluster Array(w284, w254) -> (w283:cluster{dbl, dbl}[])
    n142 = Index Array(array=w248, index=0) -> (element=w253:dbl)
    n143 = Build Cluster Array(w249, w245) -> (w246:cluster{dbl, dbl}[])
    n144 = Array Size(array=w254) -> (size(s)=w259:i32)
    n145 = Array Size(array=w245) -> (size(s)=w243:i32)
    n146 = Negate(x=w257) -> (-x=w262:dbl)
    n147 = Add(x=w262, y=w260) -> (x+y=w261:dbl)
    n148 = Select(t=w262, s=w247, f=w261) -> ()  [unwired: 1 out]
    n149 = Decrement(x=w259) -> (x-1=w256:i32)
    n150 = Negate(x=w253) -> (-x=w250:dbl)
    n151 = Add(x=w250, y=w241) -> (x+y=w251:dbl)
    n152 = Select(t=w250, s=w247, f=w251) -> ()  [unwired: 1 out]
    n153 = Decrement(x=w243) -> (x-1=w244:i32)
    n154 = Index Array(array=w254, index=w256) -> (element=w255:dbl)
    n155 = Index Array(array=w245, index=w244) -> (element=w242:dbl)
  }
  n156 = Bundle(w32) -> (w31:cluster{cluster{dbl, dbl}[]})  [unwired: 1 in]
  n157 = Bundle(w30) -> (w29:cluster{cluster{dbl, dbl}[]})  [unwired: 1 in]
  n158 = Build Array(w31, w29) -> (→"Accel":cluster{cluster{dbl, dbl}[]}[])
  n159 = Build Cluster Array(w9, w8) -> (w7:cluster{dbl, dbl}[])
  n160 = Build Cluster Array(w3, w2) -> (w4:cluster{dbl, dbl}[])
  n161 = Bundle(w27) -> (w26:cluster{cluster{dbl, dbl}[]})  [unwired: 1 in]
  n162 = Bundle(w17) -> (w24:cluster{cluster{dbl, dbl}[]})  [unwired: 1 in]
  n163 = Bundle(w20) -> ()  [unwired: 1 in, 1 out]
  n164 = Bundle(w19) -> ()  [unwired: 1 in, 1 out]
  n165 = Bundle(w7) -> (w6:cluster{cluster{dbl, dbl}[]})  [unwired: 1 in]
  n166 = Bundle(w4) -> (w1:cluster{cluster{dbl, dbl}[]})  [unwired: 1 in]
  n167 = Build Array(w23, w22, w26, w24) -> (→"VelocityProfile":cluster{cluster{"Time":dbl, "Velocity":dbl}[]}[])
  n168 = Build Array(w6, w1) -> (→"PositionProfile":cluster{cluster{dbl, dbl}[]}[])
